vi "Main[Top VI].vi"() -> ()   [LabVIEW 2011]
uses:
  <vilib>/picture/picture.llb/imagedata.ctl
panel:
  out "Trate2":dbl caption="帧率T：" format="%#.1f"
  out "Rrate2":dbl caption="帧率R：" format="%#.1f"
  out "errcnt2":i32 caption="校验错误："
  out "Trate1":dbl caption="帧率T：" format="%#.1f"
  out "DevIndex":u32
  in  "path":path
  out "Rrate1":dbl caption="帧率R：" format="%#.1f"
  out "errcnt1":i32 caption="校验错误："
  in  "reciveEnable":bool=TRUE
  in  "ID Filter Set":bool
  in  "ID Filter Str":string="01 02"
  in  "ID Filter":enum32{"enable", "disable"}(radio)=enum."disable" caption="接收滤波ID设置(直接ID号)"
  in  "list":i32(listbox)
  in  "savefile":bool
  in  "sendfile":bool
  in  "clear":bool
  in  "send stop":bool
  out "SaveCnt":u32 caption="保存总帧数:"
  in  "ID Type":enum32{"left", "right"}(radio)=enum."right" caption="ID 格式"
  in  "Send":bool
  in  "Data Inc":bool
  in  "sendcycle":i32=10 caption="发送周期:" min=0 max=99999999 step=1
  in  "data":string="00 00 00 00 00 00 00 00" caption="数据:"
  in  "ID Inc":bool
  in  "SendCnt":i32=1 caption="发送总帧数:" min=-1
  in  "CAN Channel":enum16{"1", "2"}(ring) caption="CAN通道:"
  in  "Frame ID":string="00 00 00 01" caption="帧ID:"
  in  "Frame Type":enum16{"数据帧", "远程帧"}(ring) caption="帧类型:"
  in  "Frame Format":enum16{"标准帧", "扩展帧"}(ring) caption="帧格式:"
  # "ms"
  # "统计数据：通道2"
  # "统计数据：通道1"
  # "CAN发送"
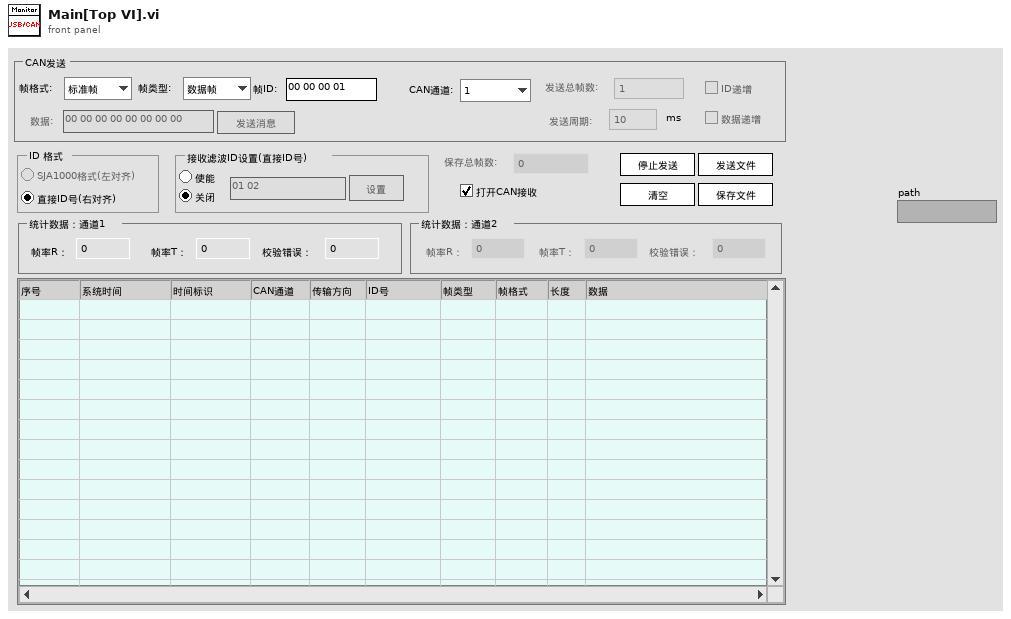
[diagram p1: front panel]
types:
  T1 = enum16{"Init", "RegistEvent", "run", "unRegistEvent", "Release", "Exit"}
  T2 = cluster{"type":u16, "scantime":u16, "highspd":bool, "disp":bool, "save":bool, "hl":bool, "ID合并":bool, "Rfun":u16, "Tfun":u16, "chk1":bool, "chk2":bool, "format":enum16{"hex", "dec", "oct", "bin"}, "rateR1":bool, "rateR2":bool, "rateT1":bool, "rateT2":bool, "RcvE1":bool, "RcvE2":bool, "TSFormat":enum16{"原始值", "实际值"}, "RcvLen":i16}
  T3 = typedef "imagedata.ctl" = cluster{"image type":i32, "image depth":i32, "image":u8[], "mask":u8[], "colors":u32[], "Rectangle":cluster{"left":i16, "top":i16, "right":i16, "bottom":i16}}
  T4 = enum8{"Enabled", "Disabled", "Disabled and Grayed Out"}
  T5 = typedef "Param.ctl" = cluster{"kCANBAUD":u8, "BTR0":u8, "BTR1":u8, "MODE":u8, "FILTER":u8, "ACR0":u32, "AMR0":u32, "FlashParam":u32, "BAUD":u32, "SJW":u8, "BRP":u8, "SAM":u8, "PHS2_SEL":u8, "PRSEG":u8, "PHSEG1":u8, "PHSEG2":u8}
  T6 = cluster{"hw_Version":u16, "fw_Version":u16, "dr_Version":u16, "in_Version":u16, "irq_Num":u16, "can_Num":u8, "str_Serial_Num":string, "str_hw_Type":string, "Reserved":u8[]}
  T7 = cluster{"hw_Version":u16, "fw_Version":u16, "dr_Version":u16, "in_Version":u16, "irq_Num":u16, "can_Num":u8, "reserved":u8, "str_Serial_Num":string, "str_hw_Type":string, "str_GYUsb_Serial":string[]}
  T8 = enum32{"Bad", "Idle", "Run top level", "Running"}
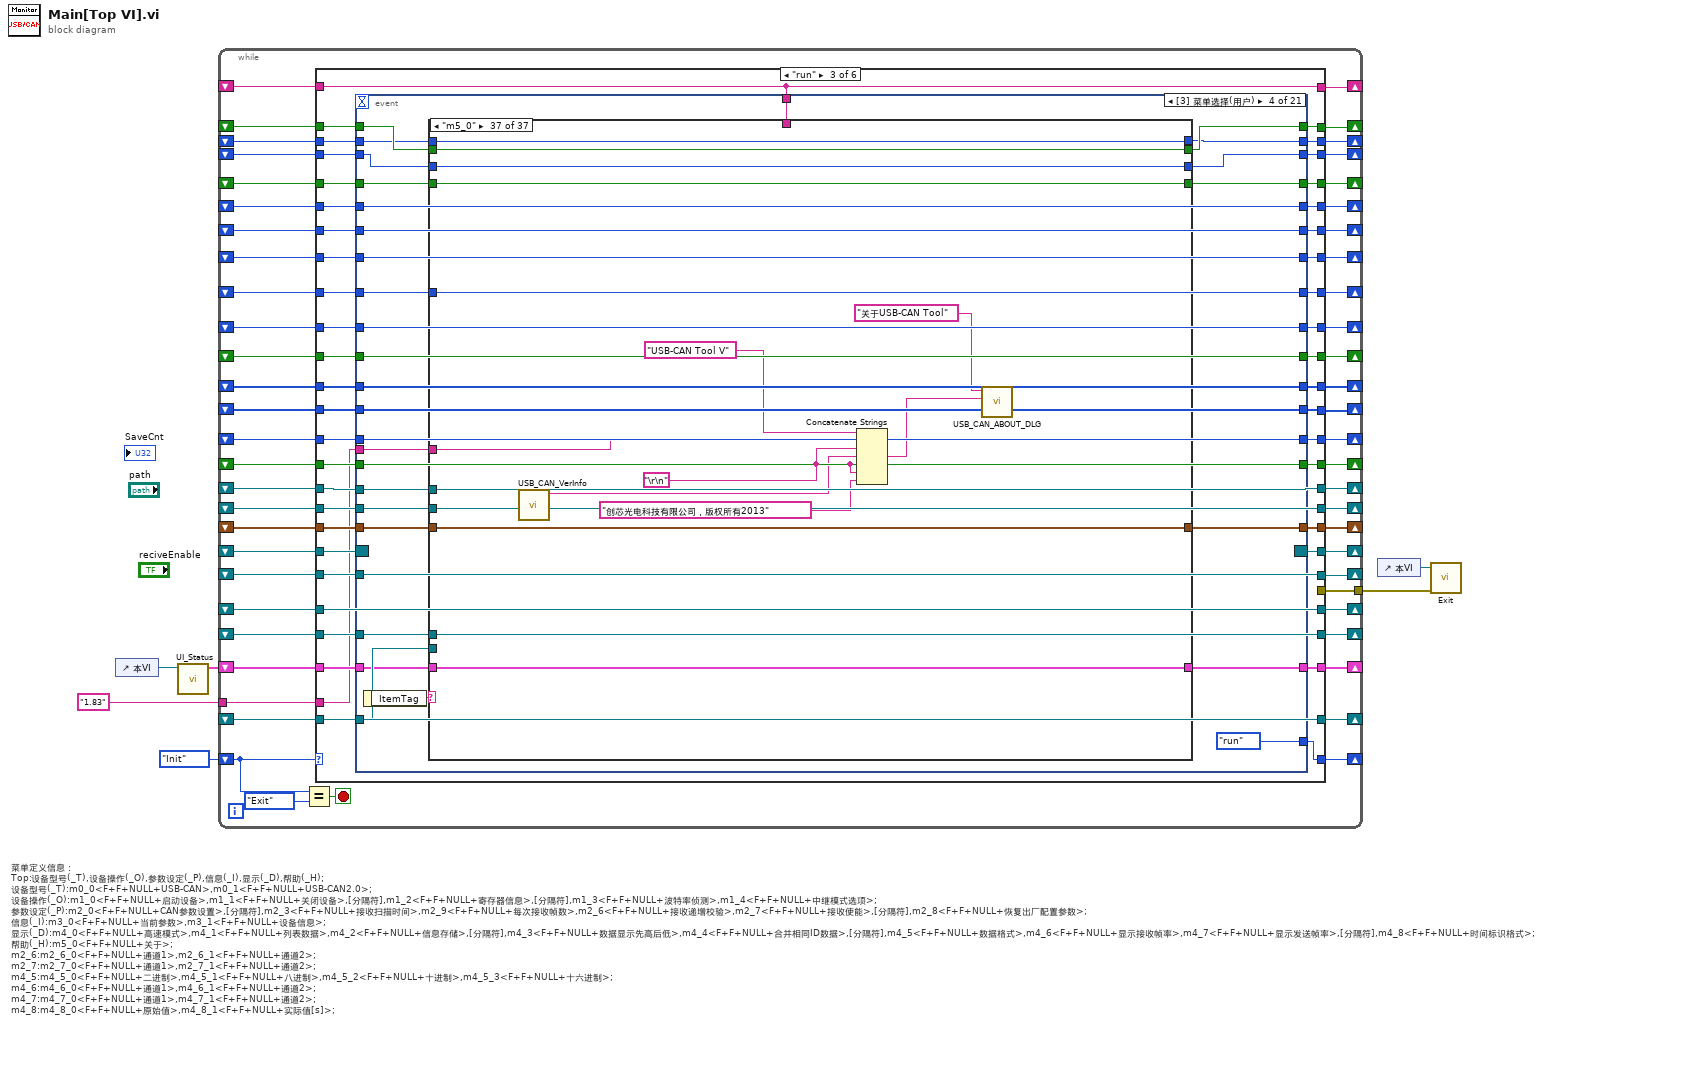
[diagram p0: block diagram]
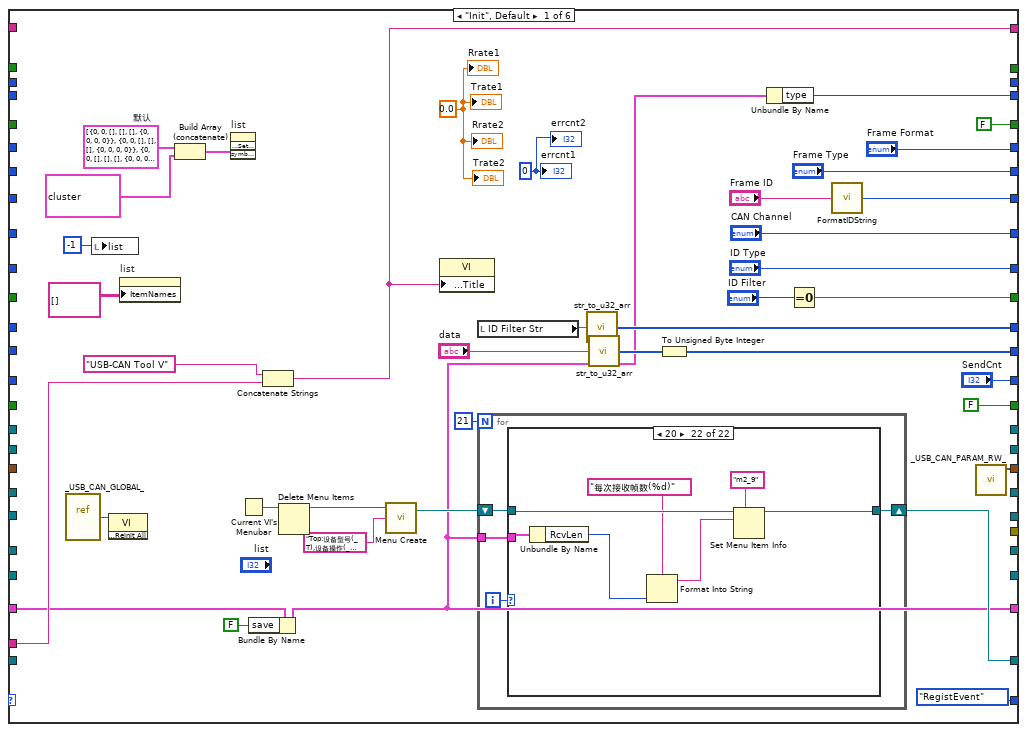
[diagram p2: hidden frame]
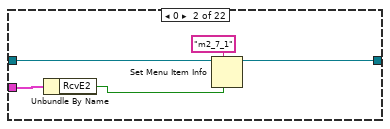
[diagram p4: hidden frame]
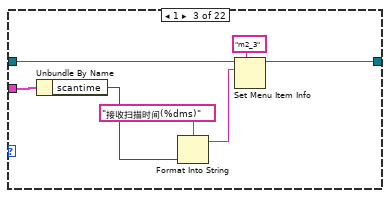
[diagram p5: hidden frame]
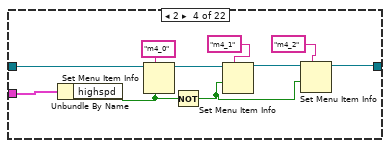
[diagram p6: hidden frame]
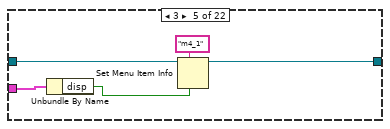
[diagram p7: hidden frame]
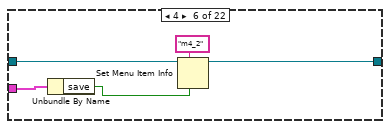
[diagram p8: hidden frame]
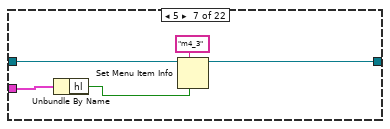
[diagram p9: hidden frame]
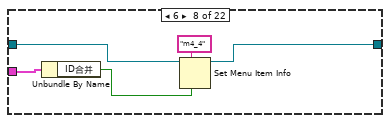
[diagram p10: hidden frame]
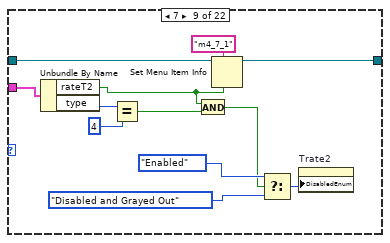
[diagram p11: hidden frame]
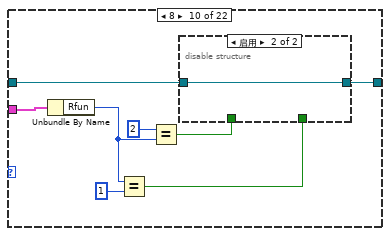
[diagram p12: hidden frame]
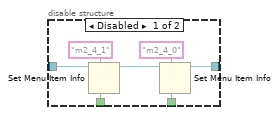
[diagram p13: hidden frame]
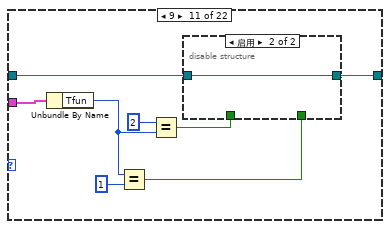
[diagram p14: hidden frame]
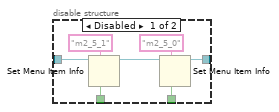
[diagram p15: hidden frame]
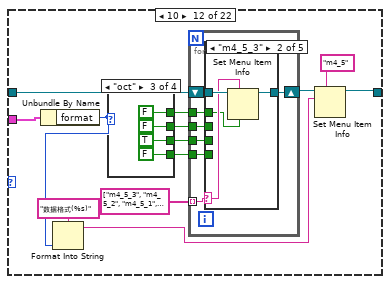
[diagram p16: hidden frame]
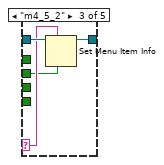
[diagram p18: hidden frame]
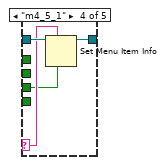
[diagram p19: hidden frame]
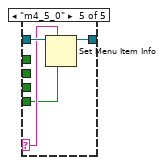
[diagram p20: hidden frame]
diagram:
  # "菜单定义信息：\nTop:设备型号(_T),设备操作(_O),参数设定(_P),信息(_I),显示(_D),帮助(_H);\n设备型号(_T):m0_0<F+F+NULL+USB-CAN>,m0_1<F+F+NULL+USB-CAN2.0>;\n设备操作(_O):m1_0<F+F+NULL+启动设备>,m1_1<F+F+NULL+关闭设备>,[分隔符],m1_2<F+F+NULL+寄存器信息>,[分隔符],m1_3<F+F+NULL+波特率侦测>,m1_4<F+F+NULL+中继模式选项>;\n参数设定(_P):m2_0<F+F+NULL+CAN参数设置>,[分隔符],m2_3<F+F+NULL+接收扫描时间>,m2_9<F+F+NULL+每次接收帧数>,m2_6<F+F+NULL+接收递增校验>,m2_7<F+F+NULL+接收使能>,[分隔符],m2_8<F+F+NULL+恢复出厂配置参数>;\n信息(_I):m3_0<F+F+NULL+当前参数>,m3_1<F+F+NULL+设备信息>;\n显示(_D):m4_0<F+F+NULL+高速模式>,m4_1<F+F+NULL+列表数据>,m4_2<F+F+NULL+信息存储>,[分隔符],m4_3<F+F+NULL+数据显示先高后低>,m4_4<F+F+NULL+合并相同ID数据>,[分隔符],m4_5<F+F+NULL+数据格式>,m4_6<F+F+NULL+显示接收帧率>,m4_7<F+F+NULL+显示发送帧率>,[分隔符],m4_8<F+F+NULL+时间标识格式>;\n帮助(_H):m5_0<F+F+NULL+关于>;\nm2_6:m2_6_0<F+F+NULL+通道1>,m2_6_1<F+F+NULL+通道2>;\nm2_7:m2_7_0<F+F+NULL+通道1>,m2_7_1<F+F+NULL+通道2>;\nm4_5:m4_5_0<F+F+NULL+二进制>,m4_5_1<F+F+NULL+八进制>,m4_5_2<F+F+NULL+十进制>,m4_5_3<F+F+NULL+十六进制>;\nm4_6:m4_6_0<F+F+NULL+通道1>,m4_6_1<F+F+NULL+通道2>;\nm4_7:m4_7_0<F+F+NULL+通道1>,m4_7_1<F+F+NULL+通道2>;\nm4_8:m4_8_0<F+F+NULL+原始值>,m4_8_1<F+F+NULL+实际值[s]>;"
  n1 = control-ref of="本VI"() -> (w5:refnum<vi>)
  n2 = call "UI_Status.vi"("VI ref"=w5) -> ("menu status in out"=w4:T2)  [unwired: 9 in, 1 out]
  n3 = while {
    shift-right: [w57] -> _
    shift-left: T1."Init" -> [w60]
    shift-right: [w56] -> _
    shift-left: _ -> [w55]
    shift-right: [w53] -> _
    shift-left: _ -> [w54]
    shift-right: [w52] -> _
    shift-left: _ -> [w51]
    shift-right: [w50] -> _
    shift-left: _ -> [w49]
    shift-right: [w48] -> _
    shift-left: _ -> [w47]
    shift-right: [w46] -> _
    shift-left: _ -> [w45]
    shift-right: [w44] -> _
    shift-left: _ -> [w43]
    shift-right: [w42] -> _
    shift-left: _ -> [w41]
    shift-right: [w40] -> _
    shift-left: _ -> [w39]
    shift-right: [w38] -> _
    shift-left: _ -> [w37]
    shift-right: [w36] -> _
    shift-left: _ -> [w35]
    shift-right: [w34] -> _
    shift-left: _ -> [w33]
    shift-right: [w31] -> _
    shift-left: _ -> [w32]
    shift-right: [w30] -> _
    shift-left: _ -> [w29]
    shift-right: [w28] -> _
    shift-left: _ -> [w27]
    shift-right: [w26] -> _
    shift-left: _ -> [w25]
    shift-right: [w24] -> _
    shift-left: _ -> [w22]
    shift-right: [w23] -> _
    shift-left: _ -> [w21]
    tunnel: [w20] -> w3
    shift-right: [w19] -> _
    shift-left: _ -> [w18]
    shift-right: [w17] -> _
    shift-left: w4 -> [w16]
    shift-right: [w15] -> _
    shift-left: _ -> [w14]
    shift-right: [w13] -> _
    shift-left: _ -> [w12]
    shift-right: [w11] -> _
    shift-left: _ -> [w10]
    shift-right: [w9] -> _
    shift-left: _ -> [w8]
    tunnel: "1.83" ("FileVersion") -> [w7]
    stop <- w58 stop-if-true
    n4 = Equal?(x=w60, y=T1."Exit") -> (x = y?=w58:bool)
    n5 = case shown="\"run\"" w60 {
      tunnel: [T1."RegistEvent" T1."run" w700 T1."Release" T1."Exit" T1."Exit"] -> w57
      tunnel: [FALSE w412 w710 _ _ _] -> w56
      tunnel: w55 -> [_ w412 w720 _ _ _]
      tunnel: w54 -> [_ w411 w719 _ _ _]
      tunnel: ["Frame Format" w411 w709 _ _ _] -> w53
      tunnel: ["Frame Type" w398 w708 _ _ _] -> w52
      tunnel: w51 -> [_ w398 w718 _ _ _]
      tunnel: [w94 w410 w707 _ _ _] -> w50
      tunnel: w49 -> [_ w410 w717 _ _ _]
      tunnel: ["CAN Channel" w397 w706 _ _ _] -> w48
      tunnel: w47 -> [_ w397 w716 _ _ _]
      tunnel: ["ID Type" w409 w705 _ _ _] -> w46
      tunnel: w45 -> [_ w409 w715 _ _ _]
      tunnel: [w64 w384 w703 _ _ _] -> w44
      tunnel: w43 -> [_ w384 w713 _ _ _]
      tunnel: [w90 w385 w704 _ _ _] -> w42
      tunnel: w41 -> [_ w385 w714 _ _ _]
      tunnel: [w81 w408 w702 _ _ _] -> w40
      tunnel: w39 -> [_ w408 w712 _ _ _]
      tunnel: ["SendCnt" w407 w701 _ _ _] -> w38
      tunnel: w37 -> [_ w407 w711 _ _ _]
      tunnel: [FALSE w406 w698 _ _ _] -> w36
      tunnel: w35 -> [_ w406 w699 _ _ _]
      tunnel: [w72 w405 w685 w2109 w2157 _] -> w34
      tunnel: w33 -> [_ w405 w685 w2109 w2157 _]
      tunnel: w32 -> [_ w404 w697 w2103 _ _]
      tunnel: [w66 w404 w696 _ _ _] -> w31
      tunnel: [_ w388 w695 _ _ _] -> w30
      tunnel: w29 -> [_ _ w695 w2127 _ _]
      tunnel: [_ w387 w694 _ _ _] -> w28
      tunnel: w27 -> [_ _ w694 w2120 _ _]
      tunnel: [w78 w399 w692 _ _ _] -> w26
      tunnel: w25 -> [_ w399 w693 w2111 _ _]
      tunnel: [_ w395 w690 _ _ _] -> w24
      tunnel: [_ w394 w689 _ _ _] -> w23
      tunnel: w22 -> [_ _ w691 w2117 _ _]
      tunnel: w21 -> [_ _ w689 w2115 _ _]
      tunnel: [_ _ _ w2114 _ _] -> w20
      tunnel: [_ w389 w688 _ _ _] -> w19
      tunnel: w18 -> [_ _ w688 w2112 _ _]
      tunnel: [w63 w380 w686 w2108 _ _] -> w17
      tunnel: w16 -> [w65 w380 w687 w2108 w2154 _]
      tunnel: [_ FALSE w683 _ _ _] -> w15
      tunnel: w14 -> [_ _ w684 _ _ _]
      tunnel: [_ w375 w682 _ _ _] -> w13
      tunnel: w12 -> [_ _ w682 w2106 _ _]
      tunnel: [_ _ w680 _ _ _] -> w11
      tunnel: w10 -> [_ _ w681 _ _ _]
      tunnel: [w69 w374 w679 w2105 w2153 w2163] -> w9
      tunnel: w8 -> [_ w374 w679 w2105 w2153 w2163]
      tunnel: w7 -> [w70 _ w678 _ _ _]
      frame "Init", Default {
        w67 = 0.0 ("rate")
        w77 = T3[] [{"image type"=0, "image depth"=0, "image"=[], "mask"=[], "colors"=[], "Rectangle"={"left"=0, "top"=0, "right"=0, "bottom"=0}}, {"image type"=0, "image depth"=0, "image"=[], "mask"=[], "colors"=[], "Rectangle"={"left"=0, "top"=0, "right"=0, "bottom"=0}}, {"image type"=0, "image depth"=0, "image"=[], "mask"=[], "colors"=[], "Rectangle"={"left"=0, "top"=0, "right"=0, "bottom"=0}}, {"image type"=0, "image depth"=0, "image"=[], "mask"=[], "colors"=[], "Rectangle"={"left"=0, "top"=0, "right"=0, "bottom"=0}}, {"image type"=0, "image depth"=0, "image"=[], "mask"=[], "colors"=[], "Rectangle"={"left"=0, "top"=0, "right"=0, "bottom"=0}}, {"image type"=0, "image depth"=0, "image"=[], "mask"=[], "colors"=[], "Rectangle"={"left"=0, "top"=0, "right"=0, "bottom"=0}}, {"image type"=0, "image depth"=0, "image"=[], "mask"=[], "colors"=[], "Rectangle"={"left"=0, "top"=0, "right"=0, "bottom"=0}}, {"image type"=0, "image depth"=0, "image"=[], "mask"=[], "colors"=[], "Rectangle"={"left"=0, "top"=0, "right"=0, "bottom"=0}}, {"image type"=0, "image depth"=0, "image"=[], "mask"=[], "colors"=[], "Rectangle"={"left"=0, "top"=0, "right"=0, "bottom"=0}}, {"image type"=0, "image depth"=0, "image"=[], "mask"=[], "colors"=[], "Rectangle"={"left"=0, "top"=0, "right"=0, "bottom"=0}}, {"image type"=0, "image depth"=0, "image"=[], "mask"=[], "colors"=[], "Rectangle"={"left"=0, "top"=0, "right"=0, "bottom"=0}}, {"image type"=0, "image depth"=0, "image"=[], "mask"=[], "colors"=[], "Rectangle"={"left"=0, "top"=0, "right"=0, "bottom"=0}}, {"image type"=0, "image depth"=0, "image"=[], "mask"=[], "colors"=[], "Rectangle"={"left"=0, "top"=0, "right"=0, "bottom"=0}}, {"image type"=0, "image depth"=0, "image"=[], "mask"=[], "colors"=[], "Rectangle"={"left"=0, "top"=0, "right"=0, "bottom"=0}}, {"image type"=0, "image depth"=0, "image"=[], "mask"=[], "colors"=[], "Rectangle"={"left"=0, "top"=0, "right"=0, "bottom"=0}}, {"image type"=0, "image depth"=0, "image"=[], "mask"=[], "colors"=[], "Rectangle"={"left"=0, "top"=0, "right"=0, "bottom"=0}}, {"image type"=0, "image depth"=0, "image"=[], "mask"=[], "colors"=[], "Rectangle"={"left"=0, "top"=0, "right"=0, "bottom"=0}}, {"image type"=0, "image depth"=0, "image"=[], "mask"=[], "colors"=[], "Rectangle"={"left"=0, "top"=0, "right"=0, "bottom"=0}}, {"image type"=0, "image depth"=0, "image"=[], "mask"=[], "colors"=[], "Rectangle"={"left"=0, "top"=0, "right"=0, "bottom"=0}}, {"image type"=0, "image depth"=0, "image"=[], "mask"=[], "colors"=[], "Rectangle"={"left"=0, "top"=0, "right"=0, "bottom"=0}}, {"image type"=0, "image depth"=0, "image"=[], "mask"=[], "colors"=[], "Rectangle"={"left"=0, "top"=0, "right"=0, "bottom"=0}}, {"image type"=0, "image depth"=0, "image"=[], "mask"=[], "colors"=[], "Rectangle"={"left"=0, "top"=0, "right"=0, "bottom"=0}}, {"image type"=0, "image depth"=0, "image"=[], "mask"=[], "colors"=[], "Rectangle"={"left"=0, "top"=0, "right"=0, "bottom"=0}}, {"image type"=0, "image depth"=0, "image"=[], "mask"=[], "colors"=[], "Rectangle"={"left"=0, "top"=0, "right"=0, "bottom"=0}}, {"image type"=0, "image depth"=0, "image"=[], "mask"=[], "colors"=[], "Rectangle"={"left"=0, "top"=0, "right"=0, "bottom"=0}}, {"image type"=0, "image depth"=0, "image"=[], "mask"=[], "colors"=[], "Rectangle"={"left"=0, "top"=0, "right"=0, "bottom"=0}}, {"image type"=0, "image depth"=0, "image"=[], "mask"=[], "colors"=[], "Rectangle"={"left"=0, "top"=0, "right"=0, "bottom"=0}}, {"image type"=0, "image depth"=0, "image"=[], "mask"=[], "colors"=[], "Rectangle"={"left"=0, "top"=0, "right"=0, "bottom"=0}}, {"image type"=0, "image depth"=0, "image"=[], "mask"=[], "colors"=[], "Rectangle"={"left"=0, "top"=0, "right"=0, "bottom"=0}}, {"image type"=0, "image depth"=0, "image"=[], "mask"=[], "colors"=[], "Rectangle"={"left"=0, "top"=0, "right"=0, "bottom"=0}}, {"image type"=0, "image depth"=0, "image"=[], "mask"=[], "colors"=[], "Rectangle"={"left"=0, "top"=0, "right"=0, "bottom"=0}}, {"image type"=0, "image depth"=0, "image"=[], "mask"=[], "colors"=[], "Rectangle"={"left"=0, "top"=0, "right"=0, "bottom"=0}}, {"image type"=0, "image depth"=0, "image"=[], "mask"=[], "colors"=[], "Rectangle"={"left"=0, "top"=0, "right"=0, "bottom"=0}}, {"image type"=0, "image depth"=0, "image"=[], "mask"=[], "colors"=[], "Rectangle"={"left"=0, "top"=0, "right"=0, "bottom"=0}}, {"image type"=0, "image depth"=0, "image"=[], "mask"=[], "colors"=[], "Rectangle"={"left"=0, "top"=0, "right"=0, "bottom"=0}}, {"image type"=0, "image depth"=0, "image"=[], "mask"=[], "colors"=[], "Rectangle"={"left"=0, "top"=0, "right"=0, "bottom"=0}}, {"image type"=0, "image depth"=0, "image"=[], "mask"=[], "colors"=[], "Rectangle"={"left"=0, "top"=0, "right"=0, "bottom"=0}}]  # 默认
        w68 = 0 ("errcnt")
        n6 = vi-ref "_USB_CAN_GLOBAL_.vi"() -> (w82:refnum<vi>)
        n7 = local write "list"(-1 ("list")) -> ()
        n8 = invoke class="VI" method="Default Vals.Reinit All"(reference=w82) -> ()  [unwired: 2 in, 3 out]
        n9 = property on="list" class="MCListbox (严格)"("ItemNames"=string[][] [] ("项名")) -> ()  [unwired: 2 in, 2 out]
        n10 = Build Array (concatenate)(w77, T3[] [{"image type"=0, "image depth"=32, "image"=array[1024 elements], "mask"=[255, 255, 255, 255, 255, 255, 255, 255, 255, 255, 255, 255, 255, 255, 255, 255, 255, 255, 255, 255, 255, 255, 255, 255, 255, 255, 255, 255, 255, 255, 255, 255], "colors"=[], "Rectangle"={"left"=0, "top"=0, "right"=16, "bottom"=16}}, {"image type"=0, "image depth"=32, "image"=array[1024 elements], "mask"=[255, 255, 255, 255, 255, 255, 255, 255, 255, 255, 255, 255, 255, 255, 255, 255, 255, 255, 255, 255, 255, 255, 255, 255, 255, 255, 255, 255, 255, 255, 255, 255], "colors"=[], "Rectangle"={"left"=0, "top"=0, "right"=16, "bottom"=16}}] ("数组")) -> (w76:T3[])
        n11 = invoke on="list" class="MCListbox (严格)" method="Custom Item Symbols.Set Symbol Array"("symbols"=w76) -> ()  [unwired: 3 in, 4 out]
        n12 = Current VI's Menubar() -> (w84:refnum<k9>)
        n13 = Bundle By Name(cluster=w65, "save"=FALSE) -> (w63:T2)
        n14 = Concatenate Strings("USB-CAN Tool V", w70) -> (w69:string)
        n15 = Delete Menu Items(9:w84) -> (3:w83:refnum<k9>)  [unwired: 1 in, 3 out]
        n16 = call "Menu Create.vi"("String"="Top:设备型号(_T),设备操作(_O),参数设定(_P),信息(_I),显示(_D),帮助(_H);\n设备型号(_T):m0_0<F+F+NULL+USB-CAN>,m0_1<F+F+NULL+USB-CAN2.0>;\n设备操作(_O):m1_0<F+F+NULL+启动设备>,m1_1<F+F+NULL+关闭设备>,[分隔符],m1_2<F+F+NULL+寄存器信息>,[分隔符],m1_3<F+F+NULL+波特率侦测>,m1_4<F+F+NULL+中继模式选项>;\n参数设定(_P):m2_0<F+F+NULL+CAN参数设置>,[分隔符],m2_3<F+F+NULL+接收扫描时间>,m2_9<F+F+NULL+每次接收帧数>,m2_6<F+F+NULL+接收递增校验>,m2_7<F+F+NULL+接收使能>,[分隔符],m2_8<F+F+NULL+恢复出厂配置参数>;\n信息(_I):m3_0<F+F+NULL+当前参数>,m3_1<F+F+NULL+设备信息>;\n显示(_D):m4_0<F+F+NULL+高速模式>,m4_1<F+F+NULL+列表数据>,m4_2<F+F+NULL+信息存储>,[分隔符],m4_3<F+F+NULL+数据显示先高后低>,m4_4<F+F+NULL+合并相同ID数据>,[分隔符],m4_5<F+F+NULL+数据格式>,m4_6<F+F+NULL+显示接收帧率>,m4_7<F+F+NULL+显示发送帧率>,[分隔符],m4_8<F+F+NULL+时间标识格式>;\n帮助(_H):m5_0<F+F+NULL+关于>;\nm2_6:m2_6_0<F+F+NULL+通道1>,m2_6_1<F+F+NULL+通道2>;\nm2_7:m2_7_0<F+F+NULL+通道1>,m2_7_1<F+F+NULL+通道2>;\nm4_5:m4_5_0<F+F+NULL+二进制>,m4_5_1<F+F+NULL+八进制>,m4_5_2<F+F+NULL+十进制>,m4_5_3<F+F+NULL+十六进制>;\nm4_6:m4_6_0<F+F+NULL+通道1>,m4_6_1<F+F+NULL+通道2>;\nm4_7:m4_7_0<F+F+NULL+通道1>,m4_7_1<F+F+NULL+通道2>;\nm4_8:m4_8_0<F+F+NULL+原始值>,m4_8_1<F+F+NULL+实际值[s]>;", "menubar in"=w83) -> ("menubar out"=w74:refnum<k9>)  [unwired: 1 in, 1 out]
        n17 = property class="VI"("Front Panel.Title"=w69) -> ()  [unwired: 2 in, 2 out]
        n18 = local read "ID Filter Str"() -> (w80:string)
        n19 = for {
          N: 21 -> [_]
          shift-right: [w100] -> w72
          shift-left: w74 -> [w101]
          tunnel: w63 -> [w102]
          i -> [w103]
          n20 = case shown="20" w103 {
            tunnel: w102 -> [_ w109 w116 w126 w131 w136 w141 w146 w158 w166 w182 w203 w251 w263 w271 w283 w291 w296 w313 _ w349 w359]
            tunnel: w101 -> [w104 w108 w115 w125 w130 w135 w140 w145 w157 w165 w181 w202 w250 w262 w270 w282 w290 w295 w311 w336 w355 w362]
            tunnel: [w104 w106 w114 w121 w129 w134 w139 w144 w155 w164 w180 w193 w248 w260 w268 w280 w288 w293 w310 w335 w351 w361] -> w100
            frame -1, Default {
            }
            frame 0 {
              n21 = Unbundle By Name(w109) -> ("RcvE2"=w105:bool)
              n22 = Set Menu Item Info(6:w105, 7:"m2_7_1" ("项标识符"), 11:w108) -> (3:w106:refnum<k9>)  [unwired: 4 in, 1 out]
            }
            frame 1 {
              n23 = Unbundle By Name(w116) -> ("scantime"=w112:u16)
              n24 = Format Into String(format string="接收扫描时间(%dms)" ("格式字符串"), w112) -> (resulting string=w110:string)  [unwired: 2 in, 1 out]
              n25 = Set Menu Item Info(7:"m2_3" ("项标识符"), 10:w110, 11:w115) -> (3:w114:refnum<k9>)  [unwired: 4 in, 1 out]
            }
            frame 2 {
              n26 = Unbundle By Name(w126) -> ("highspd"=w118:bool)
              n27 = Set Menu Item Info(6:w118, 7:"m4_0" ("项标识符"), 11:w125) -> (3:w123:refnum<k9>)  [unwired: 4 in, 1 out]
              n28 = Not(x=w118) -> (.not. x?=w117:bool)
              n29 = Set Menu Item Info(7:"m4_1" ("项标识符"), 9:w117, 11:w123) -> (3:w122:refnum<k9>)  [unwired: 4 in, 1 out]
              n30 = Set Menu Item Info(7:"m4_2" ("项标识符"), 9:w117, 11:w122) -> (3:w121:refnum<k9>)  [unwired: 4 in, 1 out]
            }
            frame 3 {
              n31 = Unbundle By Name(w131) -> ("disp"=w127:bool)
              n32 = Set Menu Item Info(6:w127, 7:"m4_1" ("项标识符"), 11:w130) -> (3:w129:refnum<k9>)  [unwired: 4 in, 1 out]
            }
            frame 4 {
              n33 = Unbundle By Name(w136) -> ("save"=w132:bool)
              n34 = Set Menu Item Info(6:w132, 7:"m4_2" ("项标识符"), 11:w135) -> (3:w134:refnum<k9>)  [unwired: 4 in, 1 out]
            }
            frame 5 {
              n35 = Unbundle By Name(w141) -> ("hl"=w137:bool)
              n36 = Set Menu Item Info(6:w137, 7:"m4_3" ("项标识符"), 11:w140) -> (3:w139:refnum<k9>)  [unwired: 4 in, 1 out]
            }
            frame 6 {
              n37 = Unbundle By Name(w146) -> ("ID合并"=w142:bool)
              n38 = Set Menu Item Info(6:w142, 7:"m4_4" ("项标识符"), 11:w145) -> (3:w144:refnum<k9>)  [unwired: 4 in, 1 out]
            }
            frame 7 {
              n39 = Unbundle By Name(w158) -> ("rateT2"=w149:bool, "type"=w151:u16)
              n40 = Equal?(x=w151, y=u16 4) -> (x = y?=w148:bool)
              n41 = And(x=w149, y=w148) -> (x .and. y?=w147:bool)
              n42 = Set Menu Item Info(6:w149, 7:"m4_7_1" ("项标识符"), 11:w157) -> (3:w155:refnum<k9>)  [unwired: 4 in, 1 out]
              n43 = Select(t=T4."Enabled" ("禁用"), s=w147, f=T4."Disabled and Grayed Out" ("禁用")) -> (s? t:f=w153:T4)
              n44 = property on="Trate2" class="DigNum (严格)"("DisabledEnum"=w153) -> ()  [unwired: 2 in, 2 out]
            }
            frame 8 {
              n45 = Unbundle By Name(w166) -> ("Rfun"=w161:u16)
              n46 = Equal?(x=w161, y=u16 1) -> (x = y?=w162:bool)
              n47 = Equal?(x=u16 2, y=w161) -> (x = y?=w159:bool)
              n48 = disable-structure shown="启用" {
                disable-tunnel: w165 -> [w173 w174]
                disable-tunnel: [w169 w174] -> w164
                disable-tunnel: w162 -> [w168 _]
                disable-tunnel: w159 -> [w167 _]
                frame Disabled {
                  n49 = Set Menu Item Info(6:w167, 7:"m2_4_1" ("项标识符"), 11:w173) -> (3:w170:refnum<k9>)  [unwired: 4 in, 1 out]
                  n50 = Set Menu Item Info(6:w168, 7:"m2_4_0" ("项标识符"), 11:w170) -> (3:w169:refnum<k9>)  [unwired: 4 in, 1 out]
                }
                frame Enabled {
                }
              }
            }
            frame 9 {
              n51 = Unbundle By Name(w182) -> ("Tfun"=w177:u16)
              n52 = Equal?(x=w177, y=u16 1) -> (x = y?=w178:bool)
              n53 = Equal?(x=u16 2, y=w177) -> (x = y?=w175:bool)
              n54 = disable-structure shown="启用" {
                disable-tunnel: w181 -> [w189 w190]
                disable-tunnel: [w185 w190] -> w180
                disable-tunnel: w178 -> [w184 _]
                disable-tunnel: w175 -> [w183 _]
                frame Disabled {
                  n55 = Set Menu Item Info(6:w183, 7:"m2_5_1" ("项标识符"), 11:w189) -> (3:w186:refnum<k9>)  [unwired: 4 in, 1 out]
                  n56 = Set Menu Item Info(6:w184, 7:"m2_5_0" ("项标识符"), 11:w186) -> (3:w185:refnum<k9>)  [unwired: 4 in, 1 out]
                }
                frame Enabled {
                }
              }
            }
            frame 10 {
              n57 = Unbundle By Name(w203) -> ("format"=w196:enum16{"hex", "dec", "oct", "bin"})
              n58 = Format Into String(format string="数据格式(%s)" ("格式字符串"), w196) -> (resulting string=w192:string)  [unwired: 2 in, 1 out]
              n59 = case shown="\"oct\"" w196 {
                tunnel: [TRUE FALSE FALSE FALSE] -> w201
                tunnel: [FALSE TRUE FALSE FALSE] -> w200
                tunnel: [FALSE FALSE TRUE FALSE] -> w199
                tunnel: [FALSE FALSE FALSE TRUE] -> w198
                frame "hex" {
                }
                frame "dec" {
                }
                frame "oct" {
                }
                frame "bin" {
                }
              }
              n60 = for {
                shift-right: [w209] -> w195
                shift-left: w202 -> [w210]
                tunnel: string[] ["m4_5_3", "m4_5_2", "m4_5_1", "m4_5_0"] -> [w208] mode=indexing
                tunnel: w201 -> [w207]
                tunnel: w200 -> [w206]
                tunnel: w199 -> [w205]
                tunnel: w198 -> [w204]
                n61 = case shown="\"m4_5_3\"" w208 {
                  selector: w208 -> [_ w213 w217 w221 w225]
                  tunnel: w210 -> [w211 w215 w219 w223 w227]
                  tunnel: [w211 w214 w218 w222 w226] -> w209
                  tunnel: w207 -> [_ w212 _ _ _]
                  tunnel: w206 -> [_ _ w216 _ _]
                  tunnel: w205 -> [_ _ _ w220 _]
                  tunnel: w204 -> [_ _ _ _ w224]
                  frame "假", Default {
                  }
                  frame "m4_5_3" {
                    n62 = Set Menu Item Info(6:w212, 7:w213, 11:w215) -> (3:w214:refnum<k9>)  [unwired: 4 in, 1 out]
                  }
                  frame "m4_5_2" {
                    n63 = Set Menu Item Info(6:w216, 7:w217, 11:w219) -> (3:w218:refnum<k9>)  [unwired: 4 in, 1 out]
                  }
                  frame "m4_5_1" {
                    n64 = Set Menu Item Info(6:w220, 7:w221, 11:w223) -> (3:w222:refnum<k9>)  [unwired: 4 in, 1 out]
                  }
                  frame "m4_5_0" {
                    n65 = Set Menu Item Info(6:w224, 7:w225, 11:w227) -> (3:w226:refnum<k9>)  [unwired: 4 in, 1 out]
                  }
                }
              }
              n66 = Set Menu Item Info(7:"m4_5" ("项标识符"), 10:w192, 11:w195) -> (3:w193:refnum<k9>)  [unwired: 4 in, 1 out]
            }
            frame 11 {
              n67 = Unbundle By Name(w251) -> ("chk1"=w244:bool)
              n68 = Set Menu Item Info(6:w244, 7:"m2_6_0" ("项标识符"), 11:w250) -> (3:w248:refnum<k9>)  [unwired: 4 in, 1 out]
              n69 = Select(t=T4."Enabled" ("禁用"), s=w244, f=T4."Disabled and Grayed Out" ("禁用")) -> (s? t:f=w246:T4)
              n70 = property on="errcnt1" class="DigNum (严格)"("DisabledEnum"=w246) -> ()  [unwired: 2 in, 2 out]
            }
            frame 12 {
              n71 = Unbundle By Name(w263) -> ("chk2"=w254:bool, "type"=w256:u16)
              n72 = Equal?(x=w256, y=u16 4) -> (x = y?=w253:bool)
              n73 = And(x=w254, y=w253) -> (x .and. y?=w252:bool)
              n74 = Set Menu Item Info(6:w254, 7:"m2_6_1" ("项标识符"), 11:w262) -> (3:w260:refnum<k9>)  [unwired: 4 in, 1 out]
              n75 = Select(t=T4."Enabled" ("禁用"), s=w252, f=T4."Disabled and Grayed Out" ("禁用")) -> (s? t:f=w258:T4)
              n76 = property on="errcnt2" class="DigNum (严格)"("DisabledEnum"=w258) -> ()  [unwired: 2 in, 2 out]
            }
            frame 13 {
              n77 = Unbundle By Name(w271) -> ("rateR1"=w264:bool)
              n78 = Set Menu Item Info(6:w264, 7:"m4_6_0" ("项标识符"), 11:w270) -> (3:w268:refnum<k9>)  [unwired: 4 in, 1 out]
              n79 = Select(t=T4."Enabled" ("禁用"), s=w264, f=T4."Disabled and Grayed Out" ("禁用")) -> (s? t:f=w266:T4)
              n80 = property on="Rrate1" class="DigNum (严格)"("DisabledEnum"=w266) -> ()  [unwired: 2 in, 2 out]
            }
            frame 14 {
              n81 = Unbundle By Name(w283) -> ("rateR2"=w274:bool, "type"=w276:u16)
              n82 = Equal?(x=w276, y=u16 4) -> (x = y?=w273:bool)
              n83 = And(x=w274, y=w273) -> (x .and. y?=w272:bool)
              n84 = Set Menu Item Info(6:w274, 7:"m4_6_1" ("项标识符"), 11:w282) -> (3:w280:refnum<k9>)  [unwired: 4 in, 1 out]
              n85 = Select(t=T4."Enabled" ("禁用"), s=w272, f=T4."Disabled and Grayed Out" ("禁用")) -> (s? t:f=w278:T4)
              n86 = property on="Rrate2" class="DigNum (严格)"("DisabledEnum"=w278) -> ()  [unwired: 2 in, 2 out]
            }
            frame 15 {
              n87 = Unbundle By Name(w291) -> ("rateT1"=w285:bool)
              n88 = Set Menu Item Info(6:w285, 7:"m4_7_0" ("项标识符"), 11:w290) -> (3:w288:refnum<k9>)  [unwired: 4 in, 1 out]
              n89 = Select(t=T4."Enabled" ("禁用"), s=w285, f=T4."Disabled and Grayed Out" ("禁用")) -> (s? t:f=w286:T4)
              n90 = property on="Trate1" class="DigNum (严格)"("DisabledEnum"=w286) -> ()  [unwired: 2 in, 2 out]
            }
            frame 16 {
              n91 = Unbundle By Name(w296) -> ("RcvE1"=w292:bool)
              n92 = Set Menu Item Info(6:w292, 7:"m2_7_0" ("项标识符"), 11:w295) -> (3:w293:refnum<k9>)  [unwired: 4 in, 1 out]
            }
            frame 17 {
              n93 = Unbundle By Name(w313) -> ("type"=w312:u16, "rateR2"=w300:bool, "rateT2"=w299:bool, "chk2"=w298:bool)
              n94 = case shown="3" w312 {
                tunnel: w311 -> [w316 w322 w334]
                tunnel: [w316 w319 w332] -> w306
                tunnel: [_ _ w331] -> w305
                tunnel: [w315 w318 w330] -> w302
                tunnel: [w315 w318 w328] -> w303
                tunnel: [w315 w318 w326] -> w301
                tunnel: w300 -> [_ _ w329]
                tunnel: w299 -> [_ _ w327]
                tunnel: w298 -> [_ _ w325]
                tunnel: [i32[] [1] ("禁用项[]") i32[] [1] ("禁用项[]") _] -> w297
                frame Default {
                  w315 = 2
                }
                frame 3 {
                  w318 = 2
                  n95 = Set Menu Item Info(6:TRUE ("已勾选"), 7:"m0_0" ("项标识符"), 11:w322) -> (3:w319:refnum<k9>)  [unwired: 4 in, 1 out]
                }
                frame 4 {
                  w323 = 2
                  w324 = 0
                  w331 = TRUE ("已勾选")
                  n96 = Set Menu Item Info(6:w331, 7:"m0_1" ("项标识符"), 11:w334) -> (3:w332:refnum<k9>)  [unwired: 4 in, 1 out]
                  n97 = Select(t=w324, s=w327, f=w323) -> (s? t:f=w328:i32)
                  n98 = Select(t=w324, s=w329, f=w323) -> (s? t:f=w330:i32)
                  n99 = Select(t=w324, s=w325, f=w323) -> (s? t:f=w326:i32)
                }
              }
              n100 = property on="CAN Channel" class="Enum (严格)"("Disabled Items []"=w297) -> ()  [unwired: 2 in, 2 out]
              n101 = property on="Trate2" class="DigNum (严格)"("DisabledEnum"=w303) -> ()  [unwired: 2 in, 2 out]
              n102 = property on="Rrate2" class="DigNum (严格)"("DisabledEnum"=w302) -> ()  [unwired: 2 in, 2 out]
              n103 = property on="errcnt2" class="DigNum (严格)"("DisabledEnum"=w301) -> ()  [unwired: 2 in, 2 out]
              n104 = Set Menu Item Info(7:"m2_6_1" ("项标识符"), 9:w305, 11:w306) -> (3:w310:refnum<k9>)  [unwired: 4 in, 1 out]
              n105 = Set Menu Item Info(7:"m2_7_1" ("项标识符"), 9:w305, 11:w306) -> ()  [unwired: 4 in, 2 out]
              n106 = Set Menu Item Info(7:"m4_6_1" ("项标识符"), 9:w305, 11:w306) -> ()  [unwired: 4 in, 2 out]
              n107 = Set Menu Item Info(7:"m4_7_1" ("项标识符"), 9:w305, 11:w306) -> ()  [unwired: 4 in, 2 out]
            }
            frame 18 {
              n108 = disable-structure shown="启用" {
                disable-tunnel: w336 -> [w343 w344]
                disable-tunnel: [w339 w344] -> w335
                frame Disabled {
                  w337 = FALSE ("已启用")
                  n109 = Set Menu Item Info(7:"m2_4" ("项标识符"), 9:w337, 11:w343) -> (0:w340:errorcluster, 3:w341:refnum<k9>)  [unwired: 4 in]
                  n110 = Set Menu Item Info(7:"m2_5" ("项标识符"), 8:w340, 9:w337, 11:w341) -> (3:w339:refnum<k9>)  [unwired: 3 in, 1 out]
                }
                frame Enabled {
                }
              }
            }
            frame 19 {
              n111 = Unbundle By Name(w349) -> ("TSFormat"=w348:enum16{"原始值", "实际值"})
              n112 = Equal?(x=w348, y=enum16{"原始值", "实际值"}."原始值") -> (x = y?=w346:bool)
              n113 = Set Menu Item Info(6:w346, 7:"m4_8_0" ("项标识符"), 11:w355) -> (0:w352:errorcluster, 3:w353:refnum<k9>)  [unwired: 4 in]
              n114 = Not(x=w346) -> (.not. x?=w345:bool)
              n115 = Set Menu Item Info(6:w345, 7:"m4_8_1" ("项标识符"), 8:w352, 11:w353) -> (3:w351:refnum<k9>)  [unwired: 3 in, 1 out]
            }
            frame 20 {
              n116 = Unbundle By Name(w359) -> ("RcvLen"=w358:i16)
              n117 = Format Into String(format string="每次接收帧数(%d)" ("格式字符串"), w358) -> (resulting string=w356:string)  [unwired: 2 in, 1 out]
              n118 = Set Menu Item Info(7:"m2_9" ("项标识符"), 10:w356, 11:w362) -> (3:w361:refnum<k9>)  [unwired: 4 in, 1 out]
            }
          }
        }
        n119 = call "str_to_u32_arr.vi"("string"=w80) -> ("array"=w64:u32[])
        n120 = call "str_to_u32_arr.vi"("string"="data") -> ("array"=w85:u32[])
        n121 = To Unsigned Byte Integer(number=w85) -> (unsigned 8bit integer=w81:u8[])
        n122 = Unbundle By Name(w63) -> ("type"=w66:u16)
        n123 = Equal To 0?(x="ID Filter") -> (x = 0?=w90:bool)
        n124 = call "FormatIDString.vi"("ID String"="Frame ID") -> ("ID"=w94:u32)
        n125 = call "_USB_CAN_PARAM_RW_.vi"() -> ("param out"=w78:T5[])  [unwired: 11 in]
        "errcnt1" <- w68
        "Rrate1" <- w67
        "Trate1" <- w67
        "errcnt2" <- w68
        "Rrate2" <- w67
        "Trate2" <- w67
      }
      frame "RegistEvent" {
        w376 = TRUE  # openCan
        w393 = TRUE  # savecancel
        w396 = TRUE  # sendover
        n126 = local read "reciveEnable"() -> (w372:bool)
        n127 = Unbundle By Name(w380) -> ("Rfun"=w379:u16, "Tfun"=w373:u16, "hl"=w371:bool, "scantime"=w367:u16)
        n128 = Open VI Reference(vi path=path "DeviceOP/ReciveThread.vi" ("VI路径")) -> (vi reference=w382:refnum<vi>, error out=w378:errorcluster)  [unwired: 5 in]
        n129 = global write "_USB_CAN_GLOBAL_.vi" "R-Enb"(w372) -> ()
        n130 = invoke class="VI" method="Ctrl Val.Set"(reference=w382, error in=w378, "Control Name"="RFun" ("控件名"), "Value"=w379) -> (reference out=w370:refnum<vi>, error out=w369:errorcluster)  [unwired: 1 in, 3 out]
        n131 = global write "_USB_CAN_GLOBAL_.vi" "Disp-HL"(w371) -> ()
        n132 = Open VI Reference(vi path=path "VIs/UpdateCANData.vi" ("VI路径"), options=0 ("选项")) -> (vi reference=w392:refnum<vi>, error out=w391:errorcluster)  [unwired: 4 in]
        n133 = Open VI Reference(vi path=path "VIs/CAN_DEBUG_Send.vi" ("VI路径")) -> (vi reference=w401:refnum<vi>, error out=w400:errorcluster)  [unwired: 5 in]
        n134 = invoke class="VI" method="Ctrl Val.Set"(reference=w370, error in=w369, "Control Name"="Scan time" ("控件名"), "Value"=w367) -> (reference out=w364:refnum<vi>, error out=w363:errorcluster)  [unwired: 1 in, 3 out]
        n135 = Create User Event(user event datatype=w393) -> (user event=w389:refnum<user-event>)  [unwired: 1 in, 1 out]
        n136 = for {
          N: 27 -> [_]
          shift-right: [w502] -> w388
          shift-left: w392 -> [w504]
          shift-right: [w501] -> _
          shift-left: w391 -> [w503]
          tunnel: w389 -> [w500]
          tunnel: w380 -> [w499]
          tunnel: w385 -> [w498]
          tunnel: w384 -> [w497]
          i -> [w505]
          n137 = case shown="25" w505 {
            tunnel: w504 -> [w507 w511 w517 w522 w529 w535 w541 w547 w554 w561 w568 w575 w581 w587 w593 w599 w606 w611 w618 w624 w630 w637 w644 w651 w658 w665 w672 w677]
            tunnel: w503 -> [w506 w510 w516 w520 w527 w534 w540 w546 w553 w560 w567 w574 w580 w586 w592 w598 w605 w609 w617 w623 w629 w636 w643 w650 w657 w664 w671 w676]
            tunnel: [w507 w508 w515 w519 w528 w533 w539 w545 w552 w559 w566 w573 w579 w585 w591 w597 w604 w608 w616 w622 w628 w635 w642 w649 w656 w663 w670 w675] -> w502
            tunnel: [w506 w509 w514 w518 w526 w532 w538 w544 w551 w558 w565 w572 w578 w584 w590 w596 w603 w607 w615 w621 w627 w634 w641 w648 w655 w662 w669 w674] -> w501
            tunnel: w500 -> [_ _ _ _ _ _ w536 _ _ _ _ _ _ _ _ _ _ _ _ _ _ _ _ _ _ _ _ _]
            tunnel: w499 -> [_ _ _ _ _ _ _ _ w549 w556 w563 w570 _ _ _ _ w601 _ _ _ _ w632 w639 w646 w653 w660 w667 _]
            tunnel: w498 -> [_ _ _ _ _ _ _ _ _ _ _ _ _ _ w588 _ _ _ _ _ _ _ _ _ _ _ _ _]
            tunnel: w497 -> [_ _ _ _ _ _ _ _ _ _ _ _ _ _ _ w594 _ _ _ _ _ _ _ _ _ _ _ _]
            frame -1, Default {
            }
            frame 0 {
              n138 = invoke class="VI" method="Default Vals.Reinit All"(reference=w511, error in=w510) -> (reference out=w508:refnum<vi>, error out=w509:errorcluster)  [unwired: 1 in, 1 out]
            }
            frame 1 {
              n139 = control-ref of="list"() -> (w512:refnum<vi>)
              n140 = invoke class="VI" method="Ctrl Val.Set"(reference=w517, error in=w516, "Control Name"="list ref" ("控件名"), "Value"=w512) -> (reference out=w515:refnum<vi>, error out=w514:errorcluster)  [unwired: 1 in, 3 out]
            }
            frame 2 {
              n141 = control-ref of="errcnt1"() -> (w521:refnum<vi>)
              n142 = invoke class="VI" method="Ctrl Val.Set"(reference=w522, error in=w520, "Control Name"="errcnt1" ("控件名"), "Value"=w521) -> (reference out=w519:refnum<vi>, error out=w518:errorcluster)  [unwired: 1 in, 3 out]
            }
            frame 3 {
              n143 = control-ref of="本VI"() -> (w524:refnum<vi>)
              n144 = invoke class="VI" method="Ctrl Val.Set"(reference=w529, error in=w527, "Control Name"="vi ref" ("控件名"), "Value"=w524) -> (reference out=w528:refnum<vi>, error out=w526:errorcluster)  [unwired: 1 in, 3 out]
            }
            frame 4 {
              n145 = control-ref of="Rrate1"() -> (w530:refnum<vi>)
              n146 = invoke class="VI" method="Ctrl Val.Set"(reference=w535, error in=w534, "Control Name"="rate0" ("控件名"), "Value"=w530) -> (reference out=w533:refnum<vi>, error out=w532:errorcluster)  [unwired: 1 in, 3 out]
            }
            frame 5 {
              n147 = invoke class="VI" method="Ctrl Val.Set"(reference=w541, error in=w540, "Control Name"="cancelEvt" ("控件名"), "Value"=w536) -> (reference out=w539:refnum<vi>, error out=w538:errorcluster)  [unwired: 1 in, 3 out]
            }
            frame 6 {
              n148 = control-ref of="path"() -> (w542:refnum<vi>)
              n149 = invoke class="VI" method="Ctrl Val.Set"(reference=w547, error in=w546, "Control Name"="path" ("控件名"), "Value"=w542) -> (reference out=w545:refnum<vi>, error out=w544:errorcluster)  [unwired: 1 in, 3 out]
            }
            frame 7 {
              n150 = Unbundle By Name(w549) -> ("chk1"=w548:bool)
              n151 = invoke class="VI" method="Ctrl Val.Set"(reference=w554, error in=w553, "Control Name"="check1" ("控件名"), "Value"=w548) -> (reference out=w552:refnum<vi>, error out=w551:errorcluster)  [unwired: 1 in, 3 out]
            }
            frame 8 {
              n152 = Unbundle By Name(w556) -> ("highspd"=w555:bool)
              n153 = invoke class="VI" method="Ctrl Val.Set"(reference=w561, error in=w560, "Control Name"="highspd" ("控件名"), "Value"=w555) -> (reference out=w559:refnum<vi>, error out=w558:errorcluster)  [unwired: 1 in, 3 out]
            }
            frame 9 {
              n154 = Unbundle By Name(w563) -> ("disp"=w562:bool)
              n155 = invoke class="VI" method="Ctrl Val.Set"(reference=w568, error in=w567, "Control Name"="disp" ("控件名"), "Value"=w562) -> (reference out=w566:refnum<vi>, error out=w565:errorcluster)  [unwired: 1 in, 3 out]
            }
            frame 10 {
              n156 = Unbundle By Name(w570) -> ("save"=w569:bool)
              n157 = invoke class="VI" method="Ctrl Val.Set"(reference=w575, error in=w574, "Control Name"="save" ("控件名"), "Value"=w569) -> (reference out=w573:refnum<vi>, error out=w572:errorcluster)  [unwired: 1 in, 3 out]
            }
            frame 11 {
              n158 = local read "reciveEnable"() -> (w576:bool)
              n159 = invoke class="VI" method="Ctrl Val.Set"(reference=w581, error in=w580, "Control Name"="Enable" ("控件名"), "Value"=w576) -> (reference out=w579:refnum<vi>, error out=w578:errorcluster)  [unwired: 1 in, 3 out]
            }
            frame 12 {
              n160 = control-ref of="SaveCnt"() -> (w582:refnum<vi>)
              n161 = invoke class="VI" method="Ctrl Val.Set"(reference=w587, error in=w586, "Control Name"="SaveCnt" ("控件名"), "Value"=w582) -> (reference out=w585:refnum<vi>, error out=w584:errorcluster)  [unwired: 1 in, 3 out]
            }
            frame 13 {
              n162 = invoke class="VI" method="Ctrl Val.Set"(reference=w593, error in=w592, "Control Name"="UseFilter" ("控件名"), "Value"=w588) -> (reference out=w591:refnum<vi>, error out=w590:errorcluster)  [unwired: 1 in, 3 out]
            }
            frame 14 {
              n163 = invoke class="VI" method="Ctrl Val.Set"(reference=w599, error in=w598, "Control Name"="Filter" ("控件名"), "Value"=w594) -> (reference out=w597:refnum<vi>, error out=w596:errorcluster)  [unwired: 1 in, 3 out]
            }
            frame 15 {
              n164 = Unbundle By Name(w601) -> ("ID合并"=w600:bool)
              n165 = invoke class="VI" method="Ctrl Val.Set"(reference=w606, error in=w605, "Control Name"="ID合并" ("控件名"), "Value"=w600) -> (reference out=w604:refnum<vi>, error out=w603:errorcluster)  [unwired: 1 in, 3 out]
            }
            frame 16 {
              n166 = control-ref of="errcnt2"() -> (w610:refnum<vi>)
              n167 = invoke class="VI" method="Ctrl Val.Set"(reference=w611, error in=w609, "Control Name"="errcnt2" ("控件名"), "Value"=w610) -> (reference out=w608:refnum<vi>, error out=w607:errorcluster)  [unwired: 1 in, 3 out]
            }
            frame 17 {
              n168 = control-ref of="Rrate2"() -> (w613:refnum<vi>)
              n169 = invoke class="VI" method="Ctrl Val.Set"(reference=w618, error in=w617, "Control Name"="rate1" ("控件名"), "Value"=w613) -> (reference out=w616:refnum<vi>, error out=w615:errorcluster)  [unwired: 1 in, 3 out]
            }
            frame 18 {
              n170 = control-ref of="Trate1"() -> (w619:refnum<vi>)
              n171 = invoke class="VI" method="Ctrl Val.Set"(reference=w624, error in=w623, "Control Name"="rate2" ("控件名"), "Value"=w619) -> (reference out=w622:refnum<vi>, error out=w621:errorcluster)  [unwired: 1 in, 3 out]
            }
            frame 19 {
              n172 = control-ref of="Trate2"() -> (w625:refnum<vi>)
              n173 = invoke class="VI" method="Ctrl Val.Set"(reference=w630, error in=w629, "Control Name"="rate3" ("控件名"), "Value"=w625) -> (reference out=w628:refnum<vi>, error out=w627:errorcluster)  [unwired: 1 in, 3 out]
            }
            frame 20 {
              n174 = Unbundle By Name(w632) -> ("chk2"=w631:bool)
              n175 = invoke class="VI" method="Ctrl Val.Set"(reference=w637, error in=w636, "Control Name"="check2" ("控件名"), "Value"=w631) -> (reference out=w635:refnum<vi>, error out=w634:errorcluster)  [unwired: 1 in, 3 out]
            }
            frame 21 {
              n176 = Unbundle By Name(w639) -> ("rateR1"=w638:bool)
              n177 = invoke class="VI" method="Ctrl Val.Set"(reference=w644, error in=w643, "Control Name"="Rrate1" ("控件名"), "Value"=w638) -> (reference out=w642:refnum<vi>, error out=w641:errorcluster)  [unwired: 1 in, 3 out]
            }
            frame 22 {
              n178 = Unbundle By Name(w646) -> ("rateR2"=w645:bool)
              n179 = invoke class="VI" method="Ctrl Val.Set"(reference=w651, error in=w650, "Control Name"="Rrate2" ("控件名"), "Value"=w645) -> (reference out=w649:refnum<vi>, error out=w648:errorcluster)  [unwired: 1 in, 3 out]
            }
            frame 23 {
              n180 = Unbundle By Name(w653) -> ("rateT1"=w652:bool)
              n181 = invoke class="VI" method="Ctrl Val.Set"(reference=w658, error in=w657, "Control Name"="Trate1" ("控件名"), "Value"=w652) -> (reference out=w656:refnum<vi>, error out=w655:errorcluster)  [unwired: 1 in, 3 out]
            }
            frame 24 {
              n182 = Unbundle By Name(w660) -> ("rateT2"=w659:bool)
              n183 = invoke class="VI" method="Ctrl Val.Set"(reference=w665, error in=w664, "Control Name"="Trate2" ("控件名"), "Value"=w659) -> (reference out=w663:refnum<vi>, error out=w662:errorcluster)  [unwired: 1 in, 3 out]
            }
            frame 26 {
              n184 = Unbundle By Name(w667) -> ("TSFormat"=w666:enum16{"原始值", "实际值"})
              n185 = invoke class="VI" method="Ctrl Val.Set"(reference=w672, error in=w671, "Control Name"="TSFormat" ("控件名"), "Value"=w666) -> (reference out=w670:refnum<vi>, error out=w669:errorcluster)  [unwired: 1 in, 3 out]
            }
            frame 25 {
              w673 = FALSE ("结束前等待")
              n186 = invoke class="VI" method="Run VI"(reference=w677, error in=w676, "Wait until done"=w673, "Auto Dispose Ref"=w673) -> (reference out=w675:refnum<vi>, error out=w674:errorcluster)  [unwired: 1 in, 3 out]
            }
          }
        }
        n187 = Close Reference(reference=w364, error in (no error)=w363) -> ()  [unwired: 1 out]
        n188 = Create User Event(user event datatype=w396) -> (user event=w394:refnum<user-event>)  [unwired: 1 in, 1 out]
        n189 = for {
          N: 12 -> [_]
          tunnel: w394 -> [w415]
          shift-right: [w418] -> w387
          shift-left: w401 -> [w419]
          shift-right: [w416] -> _
          shift-left: w400 -> [w417]
          tunnel: w373 -> [w414]
          i -> [w420]
          n190 = case shown="11" w420 {
            tunnel: w419 -> [w422 w426 w431 w437 w443 w449 w455 w461 w468 w475 w482 w490 w496]
            tunnel: [w422 w423 w428 w434 w440 w446 w452 w458 w465 w472 w479 w487 w493] -> w418
            tunnel: w417 -> [w421 w425 w430 w436 w442 w448 w454 w460 w467 w474 w481 w489 w495]
            tunnel: [w421 w424 w429 w435 w441 w447 w453 w459 w466 w473 w480 w488 w494] -> w416
            tunnel: w415 -> [_ _ w427 _ _ _ _ _ _ _ _ _ _]
            tunnel: w414 -> [_ _ _ _ _ _ _ w457 _ _ _ _ _]
            frame -1, Default {
            }
            frame 0 {
              n191 = invoke class="VI" method="Default Vals.Reinit All"(reference=w426, error in=w425) -> (reference out=w423:refnum<vi>, error out=w424:errorcluster)  [unwired: 1 in, 1 out]
            }
            frame 1 {
              n192 = invoke class="VI" method="Ctrl Val.Set"(reference=w431, error in=w430, "Control Name"="event" ("控件名"), "Value"=w427) -> (reference out=w428:refnum<vi>, error out=w429:errorcluster)  [unwired: 1 in, 3 out]
            }
            frame 2 {
              n193 = local read "sendcycle"() -> (w433:i32)
              n194 = invoke class="VI" method="Ctrl Val.Set"(reference=w437, error in=w436, "Control Name"="Cycle" ("控件名"), "Value"=w433) -> (reference out=w434:refnum<vi>, error out=w435:errorcluster)  [unwired: 1 in, 3 out]
            }
            frame 3 {
              n195 = local read "SendCnt"() -> (w439:i32)
              n196 = invoke class="VI" method="Ctrl Val.Set"(reference=w443, error in=w442, "Control Name"="FrameCnt" ("控件名"), "Value"=w439) -> (reference out=w440:refnum<vi>, error out=w441:errorcluster)  [unwired: 1 in, 3 out]
            }
            frame 4 {
              n197 = local read "ID Inc"() -> (w445:bool)
              n198 = invoke class="VI" method="Ctrl Val.Set"(reference=w449, error in=w448, "Control Name"="ID Inc" ("控件名"), "Value"=w445) -> (reference out=w446:refnum<vi>, error out=w447:errorcluster)  [unwired: 1 in, 3 out]
            }
            frame 5 {
              n199 = local read "Data Inc"() -> (w451:bool)
              n200 = invoke class="VI" method="Ctrl Val.Set"(reference=w455, error in=w454, "Control Name"="Data Inc" ("控件名"), "Value"=w451) -> (reference out=w452:refnum<vi>, error out=w453:errorcluster)  [unwired: 1 in, 3 out]
            }
            frame 10 {
              n201 = invoke class="VI" method="Ctrl Val.Set"(reference=w461, error in=w460, "Control Name"="TFun" ("控件名"), "Value"=w457) -> (reference out=w458:refnum<vi>, error out=w459:errorcluster)  [unwired: 1 in, 3 out]
            }
            frame 6 {
              n202 = local read "Frame ID"() -> (w464:string)
              n203 = call "FormatIDString.vi"("ID String"=w464) -> ("ID"=w463:u32)
              n204 = invoke class="VI" method="Ctrl Val.Set"(reference=w468, error in=w467, "Control Name"="ID" ("控件名"), "Value"=w463) -> (reference out=w465:refnum<vi>, error out=w466:errorcluster)  [unwired: 1 in, 3 out]
            }
            frame 7 {
              n205 = local read "Frame Format"() -> (w471:enum16{"标准帧", "扩展帧"})
              n206 = Not Equal To 0?(x=w471) -> (x != 0?=w470:bool)
              n207 = invoke class="VI" method="Ctrl Val.Set"(reference=w475, error in=w474, "Control Name"="ExtFrame" ("控件名"), "Value"=w470) -> (reference out=w472:refnum<vi>, error out=w473:errorcluster)  [unwired: 1 in, 3 out]
            }
            frame 8 {
              n208 = local read "Frame Type"() -> (w478:enum16{"数据帧", "远程帧"})
              n209 = Not Equal To 0?(x=w478) -> (x != 0?=w477:bool)
              n210 = invoke class="VI" method="Ctrl Val.Set"(reference=w482, error in=w481, "Control Name"="remote" ("控件名"), "Value"=w477) -> (reference out=w479:refnum<vi>, error out=w480:errorcluster)  [unwired: 1 in, 3 out]
            }
            frame 9 {
              n211 = local read "data"() -> (w485:string)
              n212 = call "str_to_u32_arr.vi"("string"=w485) -> ("array"=w486:u32[])
              n213 = To Unsigned Byte Integer(number=w486) -> (unsigned 8bit integer=w484:u8[])
              n214 = invoke class="VI" method="Ctrl Val.Set"(reference=w490, error in=w489, "Control Name"="data" ("控件名"), "Value"=w484) -> (reference out=w487:refnum<vi>, error out=w488:errorcluster)  [unwired: 1 in, 3 out]
            }
            frame 11 {
              w492 = FALSE ("结束前等待")
              n215 = invoke class="VI" method="Run VI"(reference=w496, error in=w495, "Wait until done"=w492, "Auto Dispose Ref"=w492) -> (reference out=w493:refnum<vi>, error out=w494:errorcluster)  [unwired: 1 in, 3 out]
            }
          }
        }
        n216 = Create User Event(user event datatype=w376) -> (user event=w375:refnum<user-event>)  [unwired: 1 in, 1 out]
        n217 = register-events(w394, w389, w375) -> (reference out=w395:refnum<event-registration>)  [unwired: 2 in, 1 out]
        n218 = property on="send stop" class="Bool (严格)"("Val(Sgnl)"=TRUE ("值(信号)")) -> ()  [unwired: 2 in, 2 out]
      }
      frame "run" {
        n219 = event shown="[3] 菜单选择(用户)" {
          selector: w691 -> [_ _ _ _ _ _ _ _ _ _ _ _ _ _ _ _ _ _ _ _ _]
          dyn-events: [_ _ _ _ _ _ _ _ _ _ _ _ _ _ _ _ _ _ _ _ _] -> w690
          timeout: _ -> [_ _ _ _ _ _ _ _ _ _ _ _ _ _ _ _ _ _ _ _ _]
          tunnel: w720 -> [w737 w760 w779 w794 _ w1730 w1734 w1796 w1816 w1836 w1841 w1926 w1951 w1974 w1997 w2016 w2033 w2050 w2068 w2085 w2102]
          tunnel: w719 -> [w736 w759 w778 w809 w1669 w1729 w1748 w1795 w1815 w1835 w1854 w1925 w1950 w1973 w1996 w2015 w2032 w2049 w2067 w2084 _]
          tunnel: w718 -> [w735 w758 w777 w808 w1668 w1728 w1747 w1794 w1814 w1834 w1853 w1924 w1949 w1972 w1995 w2014 w2031 w2048 w2066 _ w2101]
          tunnel: w717 -> [w734 w757 w776 w807 w1667 w1727 w1746 w1793 w1813 w1833 w1843 w1923 w1948 w1971 w1994 w2013 w2030 w2047 _ w2083 w2100]
          tunnel: w716 -> [w733 w756 w775 w795 w1659 w1726 w1731 w1792 w1812 w1832 w1837 w1922 w1947 w1970 w1993 w2012 w2029 _ w2065 w2082 w2099]
          tunnel: w715 -> [w732 w755 w774 w806 w1666 w1725 w1745 w1791 w1811 w1831 w1852 w1921 w1946 w1969 _ w2011 w2028 w2046 w2064 w2081 w2098]
          tunnel: w714 -> [w731 w754 w773 w805 w1665 w1724 w1744 w1790 w1810 w1830 w1851 w1920 w1939 _ w1992 w2010 w2027 w2045 w2063 w2080 w2097]
          tunnel: w713 -> [w730 w753 w772 w804 w1664 w1723 w1743 w1789 w1809 w1829 w1850 w1919 w1942 w1957 w1991 w2009 w2026 w2044 w2062 w2079 w2096]
          tunnel: w712 -> [w729 w752 w771 w803 w1663 w1722 w1742 w1788 w1808 w1828 w1845 w1918 w1945 w1968 w1990 _ w2025 w2043 w2061 w2078 w2095]
          tunnel: w711 -> [w728 w751 w770 w802 w1662 w1721 w1741 w1787 w1807 w1827 w1844 w1917 w1944 w1967 w1989 w2008 _ w2042 w2060 w2077 w2094]
          tunnel: [w737 w760 w779 w793 w1658 w1730 w1734 w1796 w1816 w1836 w1841 w1926 w1951 w1974 w1997 w2016 w2033 w2050 w2068 w2085 w2102] -> w710
          tunnel: [w736 w759 w778 w809 w1669 w1729 w1748 w1795 w1815 w1835 w1854 w1925 w1950 w1973 w1996 w2015 w2032 w2049 w2067 w2084 w2092] -> w709
          tunnel: [w735 w758 w777 w808 w1668 w1728 w1747 w1794 w1814 w1834 w1853 w1924 w1949 w1972 w1995 w2014 w2031 w2048 w2066 w2075 w2101] -> w708
          tunnel: [w734 w757 w776 w807 w1667 w1727 w1746 w1793 w1813 w1833 w1843 w1923 w1948 w1971 w1994 w2013 w2030 w2047 w2057 w2083 w2100] -> w707
          tunnel: [w733 w756 w775 w795 w1659 w1726 w1731 w1792 w1812 w1832 w1837 w1922 w1947 w1970 w1993 w2012 w2029 w2040 w2065 w2082 w2099] -> w706
          tunnel: [w732 w755 w774 w806 w1666 w1725 w1745 w1791 w1811 w1831 w1852 w1921 w1946 w1969 w1987 w2011 w2028 w2046 w2064 w2081 w2098] -> w705
          tunnel: [w731 w754 w773 w805 w1665 w1724 w1744 w1790 w1810 w1830 w1851 w1920 w1939 w1955 w1992 w2010 w2027 w2045 w2063 w2080 w2097] -> w704
          tunnel: [w730 w753 w772 w804 w1664 w1723 w1743 w1789 w1809 w1829 w1850 w1919 w1937 w1957 w1991 w2009 w2026 w2044 w2062 w2079 w2096] -> w703
          tunnel: [w729 w752 w771 w803 w1663 w1722 w1742 w1788 w1808 w1828 w1845 w1918 w1945 w1968 w1990 w2001 w2025 w2043 w2061 w2078 w2095] -> w702
          tunnel: [w728 w751 w770 w802 w1662 w1721 w1741 w1787 w1807 w1827 w1844 w1917 w1944 w1967 w1989 w2008 w2023 w2042 w2060 w2077 w2094] -> w701
          tunnel: [T1."run" T1."run" T1."run" T1."run" T1."run" T1."unRegistEvent" T1."run" T1."run" T1."run" T1."run" T1."run" T1."run" T1."run" T1."run" T1."run" T1."run" T1."run" T1."run" T1."run" T1."run" T1."run"] -> w700
          tunnel: w699 -> [w726 w749 w768 w800 w1660 w1719 w1739 w1785 w1805 w1825 _ _ w1941 w1960 w1986 w2006 w2022 w2039 w2056 w2074 w2091]
          tunnel: [w726 w749 w768 w800 w1660 w1719 w1739 w1785 w1805 w1825 TRUE FALSE w1941 w1960 w1986 w2006 w2022 w2039 w2056 w2074 w2091] -> w698
          tunnel: w685 -> [_ w745 _ w791 _ _ _ w1774 _ _ _ _ _ _ _ _ _ _ _ _ _]
          tunnel: w697 -> [w725 w748 w767 w799 w1647 w1717 w1738 w1784 w1804 w1824 w1847 w1912 w1940 w1959 w1985 w2005 w2021 w2038 w2055 w2073 w2090]
          tunnel: [w725 w748 w767 w798 w1647 w1717 w1738 w1784 w1804 w1824 w1847 w1912 w1940 w1959 w1985 w2005 w2021 w2038 w2055 w2073 w2090] -> w696
          tunnel: w695 -> [_ w746 _ w792 _ _ _ w1778 w1802 w1823 _ _ w1932 w1958 _ _ _ _ _ _ _]
          tunnel: w694 -> [_ _ _ w781 _ _ w1736 _ _ _ w1846 w1909 _ _ _ _ _ _ _ _ _]
          tunnel: w693 -> [w724 w738 w766 w797 w1651 w1716 w1737 w1783 w1800 w1822 w1842 w1911 w1936 w1956 w1984 w2004 w2020 w2037 w2054 w2072 w2089]
          tunnel: [w724 w738 w766 w796 w1649 w1716 w1737 w1783 w1800 w1822 w1842 w1911 w1936 w1956 w1984 w2004 w2020 w2037 w2054 w2072 w2089] -> w692
          tunnel: w689 -> [_ _ _ _ _ _ _ _ _ _ _ _ _ _ _ _ _ _ _ _ _]
          tunnel: w687 -> [w723 w743 w763 w789 w1650 w1715 w1735 w1776 w1799 w1821 w1840 w1908 w1930 w1954 w1983 w2000 w2019 w2036 w2053 w2071 w2088]
          tunnel: [w723 w741 w763 w788 w1650 w1715 w1735 w1775 w1799 w1821 w1840 w1908 w1930 w1954 w1983 w2000 w2019 w2036 w2053 w2071 w2088] -> w686
          tunnel: w684 -> [w722 w740 w762 w787 w1657 w1714 w1733 w1782 w1798 w1820 w1839 w1907 w1929 w1953 w1982 w1999 w2018 w2035 w2052 w2070 w2087]
          tunnel: [w722 w740 w762 w786 w1657 w1714 w1733 w1782 w1798 w1820 w1839 w1907 w1929 w1953 w1982 w1999 w2018 w2035 w2052 w2070 w2087] -> w683
          tunnel: w682 -> [_ _ _ w785 _ _ _ _ _ _ _ _ _ _ _ _ _ _ _ _ _]
          tunnel: w681 -> [w721 w739 w761 w784 w1644 w1713 w1732 w1781 w1797 w1819 w1838 w1906 w1928 w1952 w1981 w1998 w2017 w2034 w2051 w2069 w2086]
          tunnel: [w721 w739 w761 w783 w1648 w1713 w1732 w1781 w1797 w1819 w1838 w1906 w1928 w1952 w1981 w1998 w2017 w2034 w2051 w2069 w2086] -> w680
          tunnel: w679 -> [_ _ _ w782 w1653 _ _ _ _ _ _ _ _ _ _ _ _ _ _ _ _]
          tunnel: w678 -> [_ _ _ w780 _ _ _ _ _ _ _ _ _ _ _ _ _ _ _ _ _]
          event Timeout {
            n220 = event-data() -> ()  [unwired: 1 in, 1 out]
          }
          event User Event {
            w742 = FALSE
            n221 = event-data() -> ()  [unwired: 1 in, 1 out]
            n222 = Set Menu Item Info(6:w742, 7:"m4_2" ("项标识符"), 11:w745) -> ()  [unwired: 4 in, 2 out]
            n223 = invoke class="VI" method="Ctrl Val.Set"(reference=w746, "Control Name"="save" ("控件名"), "Value"=w742) -> ()  [unwired: 2 in, 5 out]
            n224 = Bundle By Name(cluster=w743, "save"=w742) -> (w741:T2)
          }
          event User Event {
            w764 = T4."Enabled" ("禁用")
            n225 = event-data() -> ()  [unwired: 1 in, 1 out]
            n226 = property on="send stop" class="Bool (严格)"("DisabledEnum"=T4."Disabled and Grayed Out" ("禁用")) -> ()  [unwired: 2 in, 2 out]
            n227 = property on="Send" class="Bool"("DisabledEnum"=w764) -> ()  [unwired: 2 in, 2 out]
            n228 = property on="data" class="Str"("DisabledEnum"=w764) -> ()  [unwired: 2 in, 2 out]
            n229 = property on="ID Inc" class="Bool (严格)"("DisabledEnum"=w764) -> ()  [unwired: 2 in, 2 out]
            n230 = property on="sendcycle" class="DigNum (严格)"("DisabledEnum"=w764) -> ()  [unwired: 2 in, 2 out]
            n231 = property on="Data Inc" class="Bool (严格)"("DisabledEnum"=w764) -> ()  [unwired: 2 in, 2 out]
            n232 = property on="SendCnt" class="DigNum (严格)"("DisabledEnum"=w764) -> ()  [unwired: 2 in, 2 out]
          }
          event Menu Selection (User) {
            n233 = event-data() -> ("ItemTag"=w790:string)  [unwired: 1 in]
            n234 = case shown="\"m5_0\"" w790 {
              selector: w790 -> [_ _ _ _ _ _ _ _ _ _ _ w1093 w1112 w1134 w1155 w1174 w1193 w1209 w1230 w1246 w1266 _ _ _ w1363 w1377 w1395 w1407 w1430 w1452 w1468 w1485 w1555 w1579 w1599 w1623 _]
              tunnel: w799 -> [w815 _ _ w889 w894 w925 w955 w975 w988 w1031 w1059 w1099 w1116 w1139 w1160 w1179 w1198 w1215 w1236 w1252 w1272 w1275 w1314 w1339 w1368 w1382 w1400 w1412 w1434 w1456 w1473 w1497 w1561 w1585 w1605 w1629 w1642]
              tunnel: [w815 u16 3 u16 4 w889 w894 w925 w955 w975 w988 w1031 w1059 w1099 w1116 w1139 w1160 w1179 w1198 w1215 w1236 w1252 w1272 w1275 w1314 w1339 w1368 w1382 w1400 w1412 w1434 w1456 w1473 w1497 w1561 w1585 w1605 w1629 w1642] -> w798
              tunnel: w797 -> [w814 w845 w881 w888 w896 w927 w957 w978 w990 w1032 w1061 w1101 w1118 w1137 w1158 w1177 w1196 w1213 w1234 w1250 w1270 w1276 w1321 w1341 w1367 w1381 w1399 w1411 w1433 w1455 w1472 w1496 w1559 w1583 w1603 w1627 w1641]
              tunnel: [w814 w845 w881 w888 w896 w927 w957 w978 w989 w1032 w1061 w1101 w1118 w1137 w1158 w1177 w1196 w1213 w1234 w1250 w1270 w1276 w1321 w1341 w1367 w1381 w1399 w1411 w1433 w1455 w1472 w1496 w1559 w1583 w1603 w1627 w1641] -> w796
              tunnel: w795 -> [_ _ _ _ _ _ _ _ _ w1030 _ _ _ _ _ _ _ _ _ _ _ _ _ _ _ _ _ _ _ _ _ _ _ _ _ _ _]
              tunnel: w794 -> [w813 w844 w880 w885 w895 w926 w956 _ w991 w1036 w1060 w1100 w1117 w1138 w1159 w1178 w1197 w1214 w1235 w1251 w1271 w1278 w1327 w1340 w1366 w1380 w1398 w1410 w1432 w1454 w1471 w1495 w1560 w1584 w1604 w1628 w1640]
              tunnel: [w813 w844 w880 w885 w890 w922 w952 _ w991 w1036 w1060 w1100 w1117 w1138 w1159 w1178 w1197 w1214 w1235 w1251 w1271 w1278 w1327 w1340 w1366 w1380 w1398 w1410 w1432 w1454 w1471 w1495 w1560 w1584 w1604 w1628 w1640] -> w793
              tunnel: w791 -> [_ w841 w875 _ _ _ _ _ _ _ _ w1094 w1113 w1135 w1156 w1175 w1194 w1210 w1231 w1247 w1267 _ _ _ w1365 w1379 w1397 w1409 w1431 w1453 w1470 w1486 w1556 w1580 w1600 w1624 _]
              tunnel: w792 -> [_ _ _ _ _ _ _ _ _ _ _ _ _ _ _ _ _ w1208 w1229 _ _ _ _ _ w1361 w1375 w1393 _ w1418 w1440 w1466 w1483 w1554 w1578 w1598 w1622 _]
              tunnel: w789 -> [w812 w828 w864 w887 w892 w924 w954 w977 w984 w1035 w1062 w1091 w1111 w1132 w1153 w1172 w1191 w1205 w1221 w1244 w1255 w1277 w1326 w1342 w1359 w1372 w1391 w1405 w1429 w1451 w1464 w1494 w1551 w1563 w1595 w1607 w1639]
              tunnel: [w812 w838 w874 w887 w892 w924 w954 w977 w984 w1035 w1062 w1090 w1110 w1133 w1154 w1173 w1192 w1206 w1227 w1245 w1265 w1277 w1326 w1342 w1358 w1371 w1390 w1404 w1428 w1450 w1462 w1493 w1552 w1576 w1596 w1620 w1639] -> w788
              tunnel: w787 -> [w811 w836 w872 _ _ _ _ w979 w987 w1034 w1058 w1098 w1115 w1127 w1148 w1170 w1189 w1204 w1226 w1243 w1264 w1279 w1324 w1338 w1357 w1370 w1389 w1403 w1427 w1449 w1461 w1492 w1550 w1575 w1594 w1619 w1637]
              tunnel: [w811 w836 w872 TRUE w890 w922 w952 w979 w987 w1034 w1058 w1098 w1115 w1127 w1148 w1170 w1189 w1204 w1226 w1243 w1264 w1279 w1324 w1338 w1357 w1370 w1389 w1403 w1427 w1449 w1461 w1492 w1550 w1575 w1594 w1619 w1637] -> w786
              tunnel: w785 -> [_ _ _ w884 _ _ _ _ _ _ _ _ _ _ _ _ _ _ _ _ _ _ _ _ _ _ _ _ _ _ _ _ _ _ _ _ _]
              tunnel: w784 -> [w810 w835 w871 _ _ _ _ _ w986 w1033 w1057 w1097 w1114 w1126 w1147 w1169 w1188 w1203 w1225 w1242 w1263 w1280 w1325 w1337 w1356 w1369 w1388 w1402 w1426 w1448 w1460 w1491 w1549 w1574 w1593 w1618 w1636]
              tunnel: [w810 w835 w871 _ _ _ _ _ w986 w1033 w1057 w1097 w1114 w1126 w1147 w1169 w1188 w1203 w1225 w1242 w1263 w1280 w1325 w1337 w1356 w1369 w1388 w1402 w1426 w1448 w1460 w1491 w1549 w1574 w1593 w1618 w1636] -> w783
              tunnel: w782 -> [_ _ _ _ w891 w923 w953 _ _ _ _ _ _ _ _ _ _ _ _ _ _ _ _ _ _ _ _ _ _ _ _ _ _ _ _ _ _]
              tunnel: w781 -> [_ _ _ _ _ _ _ _ w983 _ _ _ _ _ _ w1161 w1180 _ _ _ _ _ _ _ _ _ _ _ _ _ _ _ _ _ _ _ _]
              tunnel: w780 -> [_ _ _ _ _ _ _ _ _ _ _ _ _ _ _ _ _ _ _ _ _ _ _ _ _ _ _ _ _ _ _ _ _ _ _ _ w1630]
              frame "", Default {
              }
              frame "m0_0" {
                w827 = 2
                w829 = FALSE ("已勾选")
                n235 = property on="CAN Channel" class="Enum (严格)"() -> ("Value"=w825:enum16{"1", "2"})  [unwired: 2 in, 2 out]
                n236 = Set Menu Item Info(6:TRUE ("已勾选"), 7:"m0_0" ("项标识符"), 11:w841) -> (3:w840:refnum<k9>)  [unwired: 4 in, 1 out]
                n237 = Equal?(x=w825, y=enum16{"1", "2"}."2") -> (x = y?=w823:bool)
                n238 = case shown="真" w823 {
                  frame False {
                  }
                  frame True {
                    n239 = property on="CAN Channel" class="Enum (严格)"("Value"=enum16{"1", "2"}."1" ("CAN Channel")) -> ()  [unwired: 2 in, 2 out]
                  }
                }
                n240 = Set Menu Item Info(6:w829, 7:"m0_1" ("项标识符"), 11:w840) -> (3:w830:refnum<k9>)  [unwired: 4 in, 1 out]
                n241 = Set Menu Item Info(7:"m2_6_1" ("项标识符"), 9:w829, 11:w830) -> ()  [unwired: 4 in, 2 out]
                n242 = Set Menu Item Info(7:"m2_7_1" ("项标识符"), 9:w829, 11:w830) -> ()  [unwired: 4 in, 2 out]
                n243 = Set Menu Item Info(7:"m4_6_1" ("项标识符"), 9:w829, 11:w830) -> ()  [unwired: 4 in, 2 out]
                n244 = Set Menu Item Info(7:"m4_7_1" ("项标识符"), 9:w829, 11:w830) -> ()  [unwired: 4 in, 2 out]
                n245 = Open VI Reference(vi path=path "DeviceOP/ReciveThread.vi" ("VI路径")) -> (vi reference=w819:refnum<vi>, error out=w821:errorcluster)  [unwired: 5 in]
                n246 = property on="errcnt2" class="DigNum (严格)"("DisabledEnum"=w827) -> ()  [unwired: 2 in, 2 out]
                n247 = property on="Trate2" class="DigNum (严格)"("DisabledEnum"=w827) -> ()  [unwired: 2 in, 2 out]
                n248 = property on="Rrate2" class="DigNum (严格)"("DisabledEnum"=w827) -> ()  [unwired: 2 in, 2 out]
                n249 = invoke class="VI" method="Ctrl Val.Set"(reference=w819, error in=w821, "Control Name"="Enable2" ("控件名"), "Value"=FALSE) -> (reference out=w817:refnum<vi>, error out=w816:errorcluster)  [unwired: 1 in, 3 out]
                n250 = property on="CAN Channel" class="Enum (严格)"("Disabled Items []"=i32[] [1] ("禁用项[]")) -> ()  [unwired: 2 in, 2 out]
                n251 = Close Reference(reference=w817, error in (no error)=w816) -> ()  [unwired: 1 out]
                n252 = Bundle By Name(cluster=w828, "type"=u16 3 ("devtype")) -> (w838:T2)
              }
              frame "m0_1" {
                w857 = 2
                w858 = 0
                w865 = TRUE ("已勾选")
                n253 = Set Menu Item Info(6:FALSE ("已勾选"), 7:"m0_0" ("项标识符"), 11:w875) -> (3:w877:refnum<k9>)  [unwired: 4 in, 1 out]
                n254 = Unbundle By Name(w864) -> ("rateR2"=w863:bool, "rateT2"=w861:bool, "chk2"=w851:bool, "RcvE2"=w850:bool)
                n255 = Set Menu Item Info(6:w865, 7:"m0_1" ("项标识符"), 11:w877) -> (3:w866:refnum<k9>)  [unwired: 4 in, 1 out]
                n256 = Set Menu Item Info(7:"m2_6_1" ("项标识符"), 9:w865, 11:w866) -> ()  [unwired: 4 in, 2 out]
                n257 = Set Menu Item Info(7:"m2_7_1" ("项标识符"), 9:w865, 11:w866) -> ()  [unwired: 4 in, 2 out]
                n258 = Set Menu Item Info(7:"m4_6_1" ("项标识符"), 9:w865, 11:w866) -> ()  [unwired: 4 in, 2 out]
                n259 = Set Menu Item Info(7:"m4_7_1" ("项标识符"), 9:w865, 11:w866) -> ()  [unwired: 4 in, 2 out]
                n260 = Bundle By Name(cluster=w864, "type"=u16 4 ("devtype")) -> (w874:T2)
                n261 = Select(t=w858, s=w861, f=w857) -> (s? t:f=w860:i32)
                n262 = Select(t=w858, s=w863, f=w857) -> (s? t:f=w862:i32)
                n263 = Select(t=w858, s=w851, f=w857) -> (s? t:f=w859:i32)
                n264 = property on="Trate2" class="DigNum (严格)"("DisabledEnum"=w860) -> ()  [unwired: 2 in, 2 out]
                n265 = property on="errcnt2" class="DigNum (严格)"("DisabledEnum"=w859) -> ()  [unwired: 2 in, 2 out]
                n266 = property on="Rrate2" class="DigNum (严格)"("DisabledEnum"=w862) -> ()  [unwired: 2 in, 2 out]
                n267 = property on="CAN Channel" class="Enum (严格)"("Disabled Items []"=i32[] [] ("禁用项[]")) -> ()  [unwired: 2 in, 2 out]
                n268 = Open VI Reference(vi path=path "DeviceOP/ReciveThread.vi" ("VI路径")) -> (vi reference=w854:refnum<vi>, error out=w852:errorcluster)  [unwired: 5 in]
                n269 = invoke class="VI" method="Ctrl Val.Set"(reference=w854, error in=w852, "Control Name"="Enable2" ("控件名"), "Value"=w850) -> (reference out=w849:refnum<vi>, error out=w848:errorcluster)  [unwired: 1 in, 3 out]
                n270 = Close Reference(reference=w849, error in (no error)=w848) -> ()  [unwired: 1 out]
              }
              frame "m1_0" {
                n271 = Generate User Event(user event=w884, event data cluster=TRUE ("事件数据")) -> ()  [unwired: 1 in, 2 out]
              }
              frame "m1_1" {
                w890 = FALSE
                n272 = case shown="真" w895 {
                  tunnel: w894 -> [_ w899]
                  frame False {
                    n273 = call "TimeLmtDialog.vi"("Infoin"="设备已关闭！") -> ()  [unwired: 11 in]
                  }
                  frame True {
                    n274 = local read "DevIndex"() -> (w898:u32)
                    n275 = stacked-sequence {
                      tunnel: w899 -> [w901 w911]
                      tunnel: w898 -> [w900 w910]
                      frame #0 {
                        n276 = Equal?(x=w901, y=u16 4) -> (x = y?=w905:bool)
                        n277 = Select(t=2, s=w905, f=1) -> (s? t:f=w902:i32)
                        n278 = for {
                          N: w902 -> [_]
                          tunnel: w901 -> [w909]
                          tunnel: w900 -> [w908]
                          i -> [w907]
                          n279 = call "ResetCAN.vi"("CANInd"=w907, "DeciceInd"=w908, "DeviceType"=w909) -> ()  [unwired: 7 in, 2 out]
                        }
                      }
                      frame #1 {
                        n280 = call "CloseDevice.vi"("DeviceInd"=w910, "type"=w911) -> ("success"=w912:bool)  [unwired: 8 in, 1 out]
                        n281 = case shown="真" w912 {
                          frame False {
                            n282 = call "TimeLmtDialog.vi"("Infoin"="关闭失败！") -> ()  [unwired: 11 in]
                          }
                          frame True {
                            n283 = call "TimeLmtDialog.vi"("Infoin"="关闭成功！") -> ()  [unwired: 11 in]
                          }
                        }
                      }
                    }
                  }
                }
                n284 = global write "_USB_CAN_GLOBAL_.vi" "open"(FALSE ("open")) -> ()
                n285 = property class="VI"("Front Panel.Title"=w891) -> ()  [unwired: 2 in, 2 out]
              }
              frame "m1_3" {
                w922 = FALSE
                n286 = case shown="真" w926 {
                  tunnel: w925 -> [_ w929]
                  frame False {
                  }
                  frame True {
                    n287 = local read "DevIndex"() -> (w928:u32)
                    n288 = stacked-sequence {
                      tunnel: w929 -> [w931 w941]
                      tunnel: w928 -> [w930 w940]
                      frame #0 {
                        n289 = Equal?(x=w931, y=u16 4) -> (x = y?=w935:bool)
                        n290 = Select(t=2, s=w935, f=1) -> (s? t:f=w932:i32)
                        n291 = for {
                          N: w932 -> [_]
                          tunnel: w931 -> [w939]
                          tunnel: w930 -> [w938]
                          i -> [w937]
                          n292 = call "ResetCAN.vi"("CANInd"=w937, "DeciceInd"=w938, "DeviceType"=w939) -> ()  [unwired: 7 in, 2 out]
                        }
                      }
                      frame #1 {
                        n293 = call "CloseDevice.vi"("DeviceInd"=w940, "type"=w941) -> ("success"=w942:bool)  [unwired: 8 in, 1 out]
                        n294 = case shown="真" w942 {
                          frame False {
                            n295 = call "TimeLmtDialog.vi"("Infoin"="关闭失败！") -> ()  [unwired: 11 in]
                          }
                          frame True {
                            n296 = call "TimeLmtDialog.vi"("Infoin"="关闭成功！") -> ()  [unwired: 11 in]
                          }
                        }
                      }
                    }
                  }
                }
                n297 = global write "_USB_CAN_GLOBAL_.vi" "open"(FALSE ("open")) -> ()
                n298 = call "Global_Application Path.vi"() -> ("程序路径"=w918:path)  [unwired: 1 in]
                n299 = Build Path(base path=w918, name or relative path="波特率侦测.exe " ("command line")) -> (appended path=w916:path)
                n300 = Path To String(path=w916) -> (string=w915:string)
                n301 = call <vilib>:"System Exec.vi"("wait until completion? (T)"=FALSE, "command line"=w915) -> ("error out"=w919:errorcluster)  [unwired: 6 in, 3 out]
                n302 = call <vilib>:"Simple Error Handler.vi"("error in (no error)"=w919) -> ()  [unwired: 4 in, 5 out]
                n303 = property class="VI"("Front Panel.Title"=w923) -> ()  [unwired: 2 in, 2 out]
              }
              frame "m1_4" {
                w952 = FALSE
                n304 = case shown="真" w956 {
                  tunnel: w955 -> [_ w959]
                  frame False {
                  }
                  frame True {
                    n305 = local read "DevIndex"() -> (w958:u32)
                    n306 = stacked-sequence {
                      tunnel: w959 -> [w961 w971]
                      tunnel: w958 -> [w960 w970]
                      frame #0 {
                        n307 = Equal?(x=w961, y=u16 4) -> (x = y?=w965:bool)
                        n308 = Select(t=2, s=w965, f=1) -> (s? t:f=w962:i32)
                        n309 = for {
                          N: w962 -> [_]
                          tunnel: w961 -> [w969]
                          tunnel: w960 -> [w968]
                          i -> [w967]
                          n310 = call "ResetCAN.vi"("CANInd"=w967, "DeciceInd"=w968, "DeviceType"=w969) -> ()  [unwired: 7 in, 2 out]
                        }
                      }
                      frame #1 {
                        n311 = call "CloseDevice.vi"("DeviceInd"=w970, "type"=w971) -> ("success"=w972:bool)  [unwired: 8 in, 1 out]
                        n312 = case shown="真" w972 {
                          frame False {
                            n313 = call "TimeLmtDialog.vi"("Infoin"="关闭失败！") -> ()  [unwired: 11 in]
                          }
                          frame True {
                            n314 = call "TimeLmtDialog.vi"("Infoin"="关闭成功！") -> ()  [unwired: 11 in]
                          }
                        }
                      }
                    }
                  }
                }
                n315 = global write "_USB_CAN_GLOBAL_.vi" "open"(FALSE ("open")) -> ()
                n316 = call "Global_Application Path.vi"() -> ("程序路径"=w948:path)  [unwired: 1 in]
                n317 = Build Path(base path=w948, name or relative path="CANBridgeConfig.exe " ("command line")) -> (appended path=w946:path)
                n318 = Path To String(path=w946) -> (string=w945:string)
                n319 = call <vilib>:"System Exec.vi"("wait until completion? (T)"=FALSE, "command line"=w945) -> ("error out"=w949:errorcluster)  [unwired: 6 in, 3 out]
                n320 = call <vilib>:"Simple Error Handler.vi"("error in (no error)"=w949) -> ()  [unwired: 4 in, 5 out]
                n321 = property class="VI"("Front Panel.Title"=w953) -> ()  [unwired: 2 in, 2 out]
              }
              frame "m1_2" {
                n322 = global read "_USB_CAN_GLOBAL_.vi" "open"() -> (w976:bool)
                n323 = case shown="假" w976 {
                  tunnel: w975 -> [_ w982]
                  frame False {
                    n324 = call "TimeLmtDialog.vi"("Infoin"="CAN设备未打开！") -> ()  [unwired: 11 in]
                  }
                  frame True {
                    n325 = local read "DevIndex"() -> (w981:u32)
                    n326 = call "CanStatusShow.vi"("DevIndex"=w981, "DevType"=w982) -> ()  [unwired: 10 in]
                  }
                }
              }
              frame "m2_0" {
                n327 = global read "_USB_CAN_GLOBAL_.vi" "open"() -> (w985:bool)
                n328 = case shown="真" w985 {
                  selector: w985 -> [_ w998]
                  tunnel: w990 -> [w993 w997]
                  tunnel: [w993 w996] -> w989
                  tunnel: w988 -> [_ w999]
                  tunnel: w984 -> [_ w995]
                  tunnel: w983 -> [_ w994]
                  frame False {
                    n329 = call "TimeLmtDialog.vi"("Infoin"="CAN设备未打开！") -> ()  [unwired: 11 in]
                  }
                  frame True {
                    n330 = stacked-sequence {
                      tunnel: w999 -> [_ w1016 _]
                      tunnel: w998 -> [_ w1015 _]
                      tunnel: w997 -> [_ w1012 _]
                      tunnel: [_ w1011 _] -> w996
                      tunnel: w995 -> [_ _ w1027]
                      tunnel: w994 -> [w1003 _ _]
                      frame #0 {
                        w1001 = FALSE
                        n331 = invoke class="VI" method="Ctrl Val.Set"(reference=w1003, "Control Name"="Enable" ("控件名"), "Value"=w1001) -> ()  [unwired: 2 in, 5 out]
                        n332 = Open VI Reference(vi path=path "DeviceOP/ReciveThread.vi" ("VI路径")) -> (vi reference=w1004:refnum<vi>, error out=w1005:errorcluster)  [unwired: 5 in]
                        n333 = invoke class="VI" method="Ctrl Val.Set"(reference=w1004, error in=w1005, "Control Name"="Enable1" ("控件名"), "Value"=w1001) -> (reference out=w1008:refnum<vi>, error out=w1009:errorcluster)  [unwired: 1 in, 3 out]
                        n334 = Not(x=w1001) -> (.not. x?=w1000:bool)
                        n335 = invoke class="VI" method="Ctrl Val.Set"(reference=w1008, error in=w1009, "Control Name"="Enable2" ("控件名"), "Value"=w1001) -> ()  [unwired: 1 in, 5 out]
                        n336 = property on="send stop" class="Bool (严格)"("Val(Sgnl)"=w1000) -> ()  [unwired: 2 in, 2 out]
                      }
                      frame #1 {
                        n337 = local read "DevIndex"() -> (w1017:u32)
                        n338 = call "CAN-SET.vi"("DevIndex"=w1017, "open?"=w1015, "type"=w1016) -> ("success"=w1014:bool, "Param out"=w1013:T5[])  [unwired: 7 in]
                        n339 = Select(t=w1013, s=w1014, f=w1012) -> (s? t:f=w1011:T5[])
                      }
                      frame #2 {
                        n340 = Unbundle By Name(w1027) -> ("RcvE1"=w1026:bool, "RcvE2"=w1025:bool)
                        n341 = Open VI Reference(vi path=path "DeviceOP/ReciveThread.vi" ("VI路径")) -> (vi reference=w1018:refnum<vi>, error out=w1019:errorcluster)  [unwired: 5 in]
                        n342 = invoke class="VI" method="Ctrl Val.Set"(reference=w1018, error in=w1019, "Control Name"="Enable1" ("控件名"), "Value"=w1026) -> (reference out=w1022:refnum<vi>, error out=w1023:errorcluster)  [unwired: 1 in, 3 out]
                        n343 = invoke class="VI" method="Ctrl Val.Set"(reference=w1022, error in=w1023, "Control Name"="Enable2" ("控件名"), "Value"=w1025) -> ()  [unwired: 1 in, 5 out]
                      }
                    }
                  }
                }
              }
              frame "m2_1" {
                n344 = Two Button Dialog(message="是否确定恢复出厂设置？" ("消息")) -> (T button?=w1029:bool)  [unwired: 2 in]
                n345 = case shown="真" w1029 {
                  tunnel: w1031 -> [_ w1044]
                  tunnel: w1030 -> [_ _]
                  frame False {
                  }
                  frame True {
                    n346 = local read "DevIndex"() -> (w1045:u32)
                    n347 = Equal?(x=u16 4, y=w1044) -> (x = y?=w1042:bool)
                    n348 = Select(t=2, s=w1042, f=1) -> (s? t:f=w1039:i32)
                    n349 = for {
                      N: w1039 -> [_]
                      tunnel: w1045 -> [w1051]
                      tunnel: w1044 -> [w1050]
                      tunnel: [w1048] -> w1038 mode=indexing
                      i -> [w1049]
                      n350 = call "ResumeConfig.vi"("CANInd"=w1049, "DeciceInd"=w1051, "DeviceType"=w1050) -> ("Success"=w1052:bool)  [unwired: 7 in, 1 out]
                      n351 = case shown="真" w1052 {
                        tunnel: w1050 -> [_ w1056]
                        tunnel: w1051 -> [_ w1055]
                        tunnel: [_ w1054] -> w1048
                        tunnel: w1049 -> [_ w1053]
                        frame False {
                        }
                        frame True {
                          n352 = call "StartCAN.vi"("CANInd"=w1053, "DeciceInd"=w1055, "DeviceType"=w1056) -> ("Valid"=w1054:bool)  [unwired: 7 in, 1 out]
                        }
                      }
                    }
                    n353 = And Array Elements(Boolean array=w1038) -> (logical AND=w1037:bool)
                    n354 = case shown="真" w1037 {
                      frame False {
                        n355 = call "TimeLmtDialog.vi"("Infoin"="操作失败！") -> ()  [unwired: 11 in]
                      }
                      frame True {
                        n356 = call "TimeLmtDialog.vi"("Infoin"="恢复成功！") -> ()  [unwired: 11 in]
                      }
                    }
                  }
                }
              }
              frame "m2_2" {
                n357 = case shown="真" w1060 {
                  tunnel: w1059 -> [_ w1065]
                  frame False {
                    n358 = call "TimeLmtDialog.vi"("Infoin"="请先打开USB-CAN设备，再进行此操作！") -> ()  [unwired: 11 in]
                  }
                  frame True {
                    n359 = local read "DevIndex"() -> (w1064:u32)
                    n360 = call "ReadBoardInfo.vi"("DeviceInd"=w1064, "DeviceType"=w1065) -> ("VCI_BOARD_INFO"=w1066:T6, "success"=w1067:bool)  [unwired: 8 in]
                    n361 = case shown="真" w1067 {
                      tunnel: w1066 -> [_ _]
                      tunnel: w1065 -> [_ w1071]
                      tunnel: w1064 -> [_ w1070]
                      tunnel: w1064 -> [_ w1069]
                      frame False {
                        n362 = call "TimeLmtDialog.vi"("Infoin"="获取设备信息失败！") -> ()  [unwired: 11 in]
                      }
                      frame True {
                        n363 = call "_USB_CAN_BI_.vi"() -> ("change?"=w1073:bool, "BOARD_INFO out"=w1072:T7)  [unwired: 10 in]
                        n364 = case shown="真" w1073 {
                          tunnel: w1072 -> [_ w1078]
                          tunnel: w1071 -> [_ w1075]
                          tunnel: w1070 -> [_ w1077]
                          tunnel: w1069 -> [_ w1074]
                          frame False {
                          }
                          frame True {
                            n365 = call "WriteBoardInfo.vi"("BOARD_INFO"=w1078, "DeviceInd"=w1077, "DeviceType"=w1075) -> ("success"=w1076:bool)  [unwired: 8 in]
                            n366 = case shown="真" w1076 {
                              tunnel: w1075 -> [_ w1082]
                              tunnel: w1074 -> [_ w1081]
                              frame False {
                                n367 = call "TimeLmtDialog.vi"("Infoin"="修改失败！") -> ()  [unwired: 11 in]
                              }
                              frame True {
                                n368 = call "DeviceReset.vi"("DeviceInd"=w1081, "DeviceType"=w1082) -> ("Success"=w1080:bool)  [unwired: 9 in]
                                n369 = case shown="真" w1080 {
                                frame False {
                                n370 = call "TimeLmtDialog.vi"("Infoin"="修改完成，但设备重置时出错！") -> ()  [unwired: 11 in]
                                }
                                frame True {
                                n371 = call "TimeLmtDialog.vi"("Infoin"="修改成功！") -> ()  [unwired: 11 in]
                                }
                                }
                              }
                            }
                          }
                        }
                      }
                    }
                  }
                }
              }
              frame "m2_3" {
                n372 = Unbundle By Name(w1091) -> ("scantime"=w1096:u16)
                n373 = Open VI Reference(vi path=path "DeviceOP/ReciveThread.vi" ("VI路径")) -> (vi reference=w1087:refnum<vi>, error out=w1086:errorcluster)  [unwired: 5 in]
                n374 = call "Scan time Input.vi"("In"=w1096) -> ("out"=w1085:u32)  [unwired: 10 in]
                n375 = Bundle By Name(cluster=w1091, "scantime"=w1085) -> (w1090:T2)
                n376 = invoke class="VI" method="Ctrl Val.Set"(reference=w1087, error in=w1086, "Control Name"="Scan time" ("控件名"), "Value"=w1085) -> ()  [unwired: 1 in, 5 out]
                n377 = Format Into String(format string="接收扫描时间(%dms)" ("格式字符串"), w1085) -> (resulting string=w1092:string)  [unwired: 2 in, 1 out]
                n378 = Set Menu Item Info(7:w1093, 10:w1092, 11:w1094) -> ()  [unwired: 4 in, 2 out]
              }
              frame "m2_9" {
                n379 = Unbundle By Name(w1111) -> ("RcvLen"=w1109:i16)
                n380 = Open VI Reference(vi path=path "DeviceOP/ReciveThread.vi" ("VI路径")) -> (vi reference=w1104:refnum<vi>, error out=w1103:errorcluster)  [unwired: 5 in]
                n381 = call "Scan time Input.vi"("In"=w1109) -> ("out"=w1102:u32)  [unwired: 10 in]
                n382 = Bundle By Name(cluster=w1111, "RcvLen"=w1102) -> (w1110:T2)
                n383 = invoke class="VI" method="Ctrl Val.Set"(reference=w1104, error in=w1103, "Control Name"="RcvLen" ("控件名"), "Value"=w1102) -> ()  [unwired: 1 in, 5 out]
                n384 = Format Into String(format string="每次接收帧数(%d)" ("格式字符串"), w1102) -> (resulting string=w1107:string)  [unwired: 2 in, 1 out]
                n385 = Set Menu Item Info(7:w1112, 10:w1107, 11:w1113) -> ()  [unwired: 4 in, 2 out]
              }
              frame "m2_4_0" {
                n386 = Get Menu Item Info(7:w1134, 11:w1135) -> (3:w1136:refnum<k9>, 4:w1119:bool)  [unwired: 1 in, 5 out]
                n387 = Not(x=w1119) -> (.not. x?=w1125:bool)
                n388 = Set Menu Item Info(6:w1125, 7:w1134, 11:w1136) -> (3:w1121:refnum<k9>)  [unwired: 4 in, 1 out]
                n389 = Set Menu Item Info(6:w1119, 7:"m2_4_1" ("项标识符"), 11:w1121) -> ()  [unwired: 4 in, 2 out]
                n390 = Open VI Reference(vi path=path "DeviceOP/ReciveThread.vi" ("VI路径")) -> (vi reference=w1130:refnum<vi>, error out=w1128:errorcluster)  [unwired: 5 in]
                n391 = Select(t=u16 1 ("Rfun"), s=w1125, f=u16 2 ("Rfun")) -> (s? t:f=w1122:u16)
                n392 = invoke class="VI" method="Ctrl Val.Set"(reference=w1130, error in=w1128, "Control Name"="RFun" ("控件名"), "Value"=w1122) -> ()  [unwired: 1 in, 5 out]
                n393 = Bundle By Name(cluster=w1132, "Rfun"=w1122) -> (w1133:T2)
              }
              frame "m2_4_1" {
                n394 = Get Menu Item Info(7:w1155, 11:w1156) -> (3:w1157:refnum<k9>, 4:w1140:bool)  [unwired: 1 in, 5 out]
                n395 = Not(x=w1140) -> (.not. x?=w1146:bool)
                n396 = Set Menu Item Info(6:w1146, 7:w1155, 11:w1157) -> (3:w1142:refnum<k9>)  [unwired: 4 in, 1 out]
                n397 = Set Menu Item Info(6:w1140, 7:"m2_4_0" ("项标识符"), 11:w1142) -> ()  [unwired: 4 in, 2 out]
                n398 = Open VI Reference(vi path=path "DeviceOP/ReciveThread.vi" ("VI路径")) -> (vi reference=w1151:refnum<vi>, error out=w1149:errorcluster)  [unwired: 5 in]
                n399 = Select(t=u16 2 ("Rfun"), s=w1146, f=u16 1 ("Rfun")) -> (s? t:f=w1143:u16)
                n400 = invoke class="VI" method="Ctrl Val.Set"(reference=w1151, error in=w1149, "Control Name"="RFun" ("控件名"), "Value"=w1143) -> ()  [unwired: 1 in, 5 out]
                n401 = Bundle By Name(cluster=w1153, "Rfun"=w1143) -> (w1154:T2)
              }
              frame "m2_5_0" {
                n402 = Get Menu Item Info(7:w1174, 11:w1175) -> (3:w1176:refnum<k9>, 4:w1162:bool)  [unwired: 1 in, 5 out]
                n403 = Not(x=w1162) -> (.not. x?=w1168:bool)
                n404 = Set Menu Item Info(6:w1168, 7:w1174, 11:w1176) -> (3:w1164:refnum<k9>)  [unwired: 4 in, 1 out]
                n405 = Set Menu Item Info(6:w1162, 7:"m2_5_1" ("项标识符"), 11:w1164) -> ()  [unwired: 4 in, 2 out]
                n406 = Select(t=u16 1 ("Rfun"), s=w1168, f=u16 2 ("Rfun")) -> (s? t:f=w1165:u16)
                n407 = invoke class="VI" method="Ctrl Val.Set"(reference=w1161, "Control Name"="TFun" ("控件名"), "Value"=w1165) -> ()  [unwired: 2 in, 5 out]
                n408 = Bundle By Name(cluster=w1172, "Tfun"=w1165) -> (w1173:T2)
              }
              frame "m2_5_1" {
                n409 = Get Menu Item Info(7:w1193, 11:w1194) -> (3:w1195:refnum<k9>, 4:w1181:bool)  [unwired: 1 in, 5 out]
                n410 = Not(x=w1181) -> (.not. x?=w1187:bool)
                n411 = Set Menu Item Info(6:w1187, 7:w1193, 11:w1195) -> (3:w1183:refnum<k9>)  [unwired: 4 in, 1 out]
                n412 = Set Menu Item Info(6:w1181, 7:"m2_5_0" ("项标识符"), 11:w1183) -> ()  [unwired: 4 in, 2 out]
                n413 = Select(t=u16 2 ("Rfun"), s=w1187, f=u16 1 ("Rfun")) -> (s? t:f=w1184:u16)
                n414 = invoke class="VI" method="Ctrl Val.Set"(reference=w1180, "Control Name"="TFun" ("控件名"), "Value"=w1184) -> ()  [unwired: 2 in, 5 out]
                n415 = Bundle By Name(cluster=w1191, "Tfun"=w1184) -> (w1192:T2)
              }
              frame "m2_6_0" {
                n416 = Get Menu Item Info(7:w1209, 11:w1210) -> (3:w1212:refnum<k9>, 4:w1211:bool)  [unwired: 1 in, 5 out]
                n417 = Not(x=w1211) -> (.not. x?=w1202:bool)
                n418 = Set Menu Item Info(6:w1202, 7:w1209, 11:w1212) -> ()  [unwired: 4 in, 2 out]
                n419 = invoke class="VI" method="Ctrl Val.Set"(reference=w1208, "Control Name"="check1" ("控件名"), "Value"=w1202) -> ()  [unwired: 2 in, 5 out]
                n420 = Select(t=T4."Enabled" ("禁用"), s=w1202, f=T4."Disabled and Grayed Out" ("禁用")) -> (s? t:f=w1199:T4)
                n421 = Bundle By Name(cluster=w1205, "chk1"=w1202) -> (w1206:T2)
                n422 = property on="errcnt1" class="DigNum (严格)"("DisabledEnum"=w1199) -> ()  [unwired: 2 in, 2 out]
              }
              frame "m2_6_1" {
                n423 = Get Menu Item Info(7:w1230, 11:w1231) -> (3:w1233:refnum<k9>, 4:w1232:bool)  [unwired: 1 in, 5 out]
                n424 = Not(x=w1232) -> (.not. x?=w1217:bool)
                n425 = Set Menu Item Info(6:w1217, 7:w1230, 11:w1233) -> ()  [unwired: 4 in, 2 out]
                n426 = Unbundle By Name(w1221) -> ("type"=w1220:u16)
                n427 = Equal?(x=u16 4, y=w1220) -> (x = y?=w1218:bool)
                n428 = And(x=w1218, y=w1217) -> (x .and. y?=w1216:bool)
                n429 = Bundle By Name(cluster=w1221, "chk2"=w1217) -> (w1227:T2)
                n430 = invoke class="VI" method="Ctrl Val.Set"(reference=w1229, "Control Name"="check2" ("控件名"), "Value"=w1216) -> ()  [unwired: 2 in, 5 out]
                n431 = Select(t=T4."Enabled" ("禁用"), s=w1216, f=T4."Disabled and Grayed Out" ("禁用")) -> (s? t:f=w1222:T4)
                n432 = property on="errcnt2" class="DigNum (严格)"("DisabledEnum"=w1222) -> ()  [unwired: 2 in, 2 out]
              }
              frame "m2_7_0" {
                n433 = Get Menu Item Info(7:w1246, 11:w1247) -> (3:w1249:refnum<k9>, 4:w1248:bool)  [unwired: 1 in, 5 out]
                n434 = Not(x=w1248) -> (.not. x?=w1237:bool)
                n435 = Set Menu Item Info(6:w1237, 7:w1246, 11:w1249) -> ()  [unwired: 4 in, 2 out]
                n436 = Open VI Reference(vi path=path "DeviceOP/ReciveThread.vi" ("VI路径")) -> (vi reference=w1240:refnum<vi>, error out=w1238:errorcluster)  [unwired: 5 in]
                n437 = invoke class="VI" method="Ctrl Val.Set"(reference=w1240, error in=w1238, "Control Name"="Enable1" ("控件名"), "Value"=w1237) -> ()  [unwired: 1 in, 5 out]
                n438 = Bundle By Name(cluster=w1244, "RcvE1"=w1237) -> (w1245:T2)
              }
              frame "m2_7_1" {
                n439 = Get Menu Item Info(7:w1266, 11:w1267) -> (3:w1269:refnum<k9>, 4:w1268:bool)  [unwired: 1 in, 5 out]
                n440 = Not(x=w1268) -> (.not. x?=w1254:bool)
                n441 = Set Menu Item Info(6:w1254, 7:w1266, 11:w1269) -> ()  [unwired: 4 in, 2 out]
                n442 = Unbundle By Name(w1255) -> ("type"=w1258:u16)
                n443 = Open VI Reference(vi path=path "DeviceOP/ReciveThread.vi" ("VI路径")) -> (vi reference=w1261:refnum<vi>, error out=w1259:errorcluster)  [unwired: 5 in]
                n444 = Equal?(x=u16 4, y=w1258) -> (x = y?=w1256:bool)
                n445 = And(x=w1256, y=w1254) -> (x .and. y?=w1253:bool)
                n446 = invoke class="VI" method="Ctrl Val.Set"(reference=w1261, error in=w1259, "Control Name"="Enable2" ("控件名"), "Value"=w1253) -> ()  [unwired: 1 in, 5 out]
                n447 = Bundle By Name(cluster=w1255, "RcvE2"=w1253) -> (w1265:T2)
              }
              frame "m2_8" {
                # "恢复出厂设置（软件参数重置）"
                n448 = Two Button Dialog(message="本操作将重置软件参数至初始状态。\n重置后将导致当前软件界面设置、CAN配置参数等丢失！\n重置后，重启本软件生效，是否确定重置？" ("消息")) -> (T button?=w1273:bool)  [unwired: 2 in]
                n449 = case shown="真" w1273 {
                  tunnel: w1275 -> [_ w1281]
                  frame False {
                  }
                  frame True {
                    n450 = stacked-sequence {
                      tunnel: w1281 -> [_ _ w1303 _ _]
                      frame #0 {
                        n451 = call "Global_Application Path.vi"() -> ("程序路径"=w1284:path)  [unwired: 1 in]
                        n452 = Build Path(base path=w1284, name or relative path="usb_can.ini" ("名称或相对路径")) -> (appended path=w1283:path)
                        n453 = Delete(path (use dialog)=w1283) -> (error out=w1282:errorcluster)  [unwired: 4 in, 2 out]
                        n454 = call <vilib>:"Clear Errors.vi"("error in (no error)"=w1282) -> ()  [unwired: 6 in, 1 out]
                      }
                      frame #1 {
                        n455 = property class="VI"() -> ("Name"=w1292:string)  [unwired: 2 in, 2 out]
                        n456 = call "Global_Application Path.vi"() -> ("程序路径"=w1289:path)  [unwired: 1 in]
                        n457 = String To Byte Array(string=w1292) -> (unsigned byte array=w1291:u8[])
                        n458 = for {
                          N: 4 -> [_]
                          tunnel: w1291 -> [w1301] mode=indexing
                          shift-right: [w1298] -> w1293
                          shift-left: "" -> [w1299]
                          n459 = Format Into String(format string="%02x" ("格式字符串"), initial string=w1299, w1301) -> (resulting string=w1298:string)  [unwired: 1 in, 1 out]
                        }
                        n460 = String Subset(string=w1293, length (rest)=16 ("长度（剩余）")) -> (substring=w1295:string)  [unwired: 1 in]
                        n461 = Concatenate Strings(w1295, ".uis" ("字符串")) -> (w1288:string)
                        n462 = Build Path(base path=w1289, name or relative path=w1288) -> (appended path=w1287:path)
                        n463 = Delete(path (use dialog)=w1287) -> (error out=w1286:errorcluster)  [unwired: 4 in, 2 out]
                        n464 = call <vilib>:"Clear Errors.vi"("error in (no error)"=w1286) -> ()  [unwired: 6 in, 1 out]
                      }
                      frame #2 {
                        n465 = local read "DevIndex"() -> (w1302:u32)
                        n466 = call "CloseDevice.vi"("DeviceInd"=w1302, "type"=w1303) -> ()  [unwired: 8 in, 2 out]
                      }
                      frame #3 {
                        n467 = call "Global_Application Path.vi"() -> ("程序路径"=w1310:path)  [unwired: 1 in]
                        n468 = call "Global_Application Path.vi"("Use ExeFilePath"=TRUE) -> ("程序路径"=w1309:path)
                        n469 = Path To String(path=w1309) -> (string=w1307:string)
                        n470 = Concatenate Strings("reboot.exe -- run \"" ("command line"), w1307, "\" w:4000 \"t:USB_CAN Tool -- Reboot\"" ("字符串")) -> (w1306:string)
                        n471 = call <vilib>:"System Exec.vi"("wait until completion? (T)"=FALSE, "working directory"=w1310, "command line"=w1306) -> ("error out"=w1311:errorcluster)  [unwired: 5 in, 3 out]
                        n472 = call <vilib>:"Clear Errors.vi"("error in (no error)"=w1311) -> ()  [unwired: 6 in, 1 out]
                      }
                      frame #4 {
                        n473 = control-ref of="本VI"() -> (w1313:refnum<vi>)
                        n474 = call "Exit.vi"("VI引用"=w1313) -> ()  [unwired: 10 in, 1 out]
                      }
                    }
                  }
                }
              }
              frame "m3_0" {
                n475 = Equal?(x=w1314, y=u16 4) -> (x = y?=w1318:bool)
                n476 = Select(t=2, s=w1318, f=1) -> (s? t:f=w1315:i32)
                n477 = for {
                  N: w1315 -> [_]
                  tunnel: w1314 -> [w1333]
                  tunnel: [w1331] -> w1323 mode=indexing
                  tunnel: [w1330] -> w1320 mode=indexing
                  i -> [w1328]
                  w1329 = u32 15 items=["REFTYPE_MODE"=0, "REFTYPE_FILTER"=1, "REFTYPE_ACR0"=2, "REFTYPE_AMR0"=6, "REFTYPE_kCANBAUD"=10, "REFTYPE_CANRX_EN"=13, "REFTYPE_UARTBAUD"=14, "REFTYPE_ALL"=15] ("RefType")
                  n478 = local read "DevIndex"() -> (w1332:u32)
                  n479 = call "GetReference2.vi"("DeviceType"=w1333, "DeviceInd"=w1332, "CANInd"=w1328, "RefType"=w1329) -> ("Success"=w1331:bool, "Param"=w1330:T5)  [unwired: 9 in, 1 out]
                }
                n480 = And Array Elements(Boolean array=w1323) -> (logical AND=w1322:bool)
                n481 = case shown="真" w1322 {
                  tunnel: w1320 -> [_ w1336]
                  tunnel: w1314 -> [_ w1335]
                  frame False {
                    n482 = call "TimeLmtDialog.vi"("Infoin"="获取失败！") -> ()  [unwired: 11 in]
                  }
                  frame True {
                    n483 = call "CAN_ParamShow.vi"("DevType"=w1335, "param"=w1336) -> ()  [unwired: 10 in]
                  }
                }
              }
              frame "m3_1" {
                n484 = case shown="真" w1340 {
                  tunnel: w1339 -> [_ w1347]
                  frame False {
                    n485 = call "TimeLmtDialog.vi"("Infoin"="请先打开USB-CAN设备，再进行此操作！") -> ()  [unwired: 11 in]
                  }
                  frame True {
                    n486 = local read "DevIndex"() -> (w1346:u32)
                    n487 = call "ReadBoardInfo.vi"("DeviceInd"=w1346, "DeviceType"=w1347) -> ("VCI_BOARD_INFO"=w1344:T6, "success"=w1345:bool)  [unwired: 8 in]
                    n488 = case shown="真" w1345 {
                      tunnel: w1344 -> [_ w1349]
                      frame False {
                        n489 = call "TimeLmtDialog.vi"("Infoin"="读取失败！") -> ()  [unwired: 11 in]
                      }
                      frame True {
                        n490 = call "_USB_CAN_BOARD_INFO_.vi"("VCI_BOARD_INFO"=w1349) -> ()  [unwired: 11 in]
                      }
                    }
                  }
                }
              }
              frame "m4_0" {
                n491 = Get Menu Item Info(7:w1363, 11:w1365) -> (3:w1364:refnum<k9>, 4:w1362:bool)  [unwired: 1 in, 5 out]
                n492 = Not(x=w1362) -> (.not. x?=w1351:bool)
                n493 = Set Menu Item Info(6:w1351, 7:w1363, 11:w1364) -> (3:w1352:refnum<k9>)  [unwired: 4 in, 1 out]
                n494 = invoke class="VI" method="Ctrl Val.Set"(reference=w1361, "Control Name"="highspd" ("控件名"), "Value"=w1351) -> ()  [unwired: 2 in, 5 out]
                n495 = Not(x=w1351) -> (.not. x?=w1350:bool)
                n496 = Set Menu Item Info(7:"m4_1" ("项标识符"), 9:w1350, 11:w1352) -> (3:w1355:refnum<k9>)  [unwired: 4 in, 1 out]
                n497 = Set Menu Item Info(7:"m4_2" ("项标识符"), 9:w1350, 11:w1355) -> ()  [unwired: 4 in, 2 out]
                n498 = Bundle By Name(cluster=w1359, "highspd"=w1351) -> (w1358:T2)
              }
              frame "m4_1" {
                n499 = Get Menu Item Info(7:w1377, 11:w1379) -> (3:w1378:refnum<k9>, 4:w1376:bool)  [unwired: 1 in, 5 out]
                n500 = Not(x=w1376) -> (.not. x?=w1373:bool)
                n501 = Set Menu Item Info(6:w1373, 7:w1377, 11:w1378) -> ()  [unwired: 4 in, 2 out]
                n502 = invoke class="VI" method="Ctrl Val.Set"(reference=w1375, "Control Name"="disp" ("控件名"), "Value"=w1373) -> ()  [unwired: 2 in, 5 out]
                n503 = Bundle By Name(cluster=w1372, "disp"=w1373) -> (w1371:T2)
              }
              frame "m4_2" {
                n504 = Get Menu Item Info(7:w1395, 11:w1397) -> (3:w1396:refnum<k9>, 4:w1394:bool)  [unwired: 1 in, 5 out]
                n505 = Not(x=w1394) -> (.not. x?=w1383:bool)
                n506 = Set Menu Item Info(6:w1383, 7:w1395, 11:w1396) -> ()  [unwired: 4 in, 2 out]
                n507 = invoke class="VI" method="Ctrl Val.Set"(reference=w1393, "Control Name"="save" ("控件名"), "Value"=w1383) -> (reference out=w1386:refnum<vi>, error out=w1385:errorcluster)  [unwired: 2 in, 3 out]
                n508 = Bundle By Name(cluster=w1391, "save"=w1383) -> (w1390:T2)
                n509 = invoke class="VI" method="Ctrl Val.Set"(reference=w1386, error in=w1385, "Control Name"="sPth_Sel" ("控件名"), "Value"=w1383) -> ()  [unwired: 1 in, 5 out]
                n510 = property on="path" class="Path"("Value"=path "" ("path")) -> ()  [unwired: 2 in, 2 out]
              }
              frame "m4_3" {
                n511 = Get Menu Item Info(7:w1407, 11:w1409) -> (3:w1408:refnum<k9>, 4:w1406:bool)  [unwired: 1 in, 5 out]
                n512 = Not(x=w1406) -> (.not. x?=w1401:bool)
                n513 = Set Menu Item Info(6:w1401, 7:w1407, 11:w1408) -> ()  [unwired: 4 in, 2 out]
                n514 = global write "_USB_CAN_GLOBAL_.vi" "Disp-HL"(w1401) -> ()
                n515 = Bundle By Name(cluster=w1405, "hl"=w1401) -> (w1404:T2)
              }
              frame "m4_8_0" {
                n516 = Get Menu Item Info(7:w1430, 11:w1431) -> (3:w1425:refnum<k9>, 4:w1423:bool)  [unwired: 1 in, 5 out]
                n517 = Set Menu Item Info(6:w1423, 7:"m4_8_1" ("项标识符"), 11:w1425) -> (3:w1422:refnum<k9>)  [unwired: 4 in, 1 out]
                n518 = Not(x=w1423) -> (.not. x?=w1421:bool)
                n519 = Set Menu Item Info(6:w1421, 7:w1430, 11:w1422) -> ()  [unwired: 4 in, 2 out]
                n520 = Select(t=enum16{"原始值", "实际值"}."原始值" ("TSFormat"), s=w1421, f=enum16{"原始值", "实际值"}."实际值" ("TSFormat")) -> (s? t:f=w1417:enum16{"原始值", "实际值"})
                n521 = invoke class="VI" method="Ctrl Val.Set"(reference=w1418, "Control Name"="TSFormat" ("控件名"), "Value"=w1417) -> (reference out=w1413:refnum<vi>)  [unwired: 2 in, 4 out]
                n522 = Bundle By Name(cluster=w1429, "TSFormat"=w1417) -> (w1428:T2)
                n523 = invoke class="VI" method="Ctrl Val.Set"(reference=w1413, "Control Name"="ForceUpt" ("控件名"), "Value"=TRUE) -> ()  [unwired: 2 in, 5 out]
              }
              frame "m4_8_1" {
                n524 = Get Menu Item Info(7:w1452, 11:w1453) -> (3:w1447:refnum<k9>, 4:w1445:bool)  [unwired: 1 in, 5 out]
                n525 = Set Menu Item Info(6:w1445, 7:"m4_8_0" ("项标识符"), 11:w1447) -> (3:w1444:refnum<k9>)  [unwired: 4 in, 1 out]
                n526 = Not(x=w1445) -> (.not. x?=w1443:bool)
                n527 = Set Menu Item Info(6:w1443, 7:w1452, 11:w1444) -> ()  [unwired: 4 in, 2 out]
                n528 = Select(t=enum16{"原始值", "实际值"}."实际值" ("TSFormat"), s=w1443, f=enum16{"原始值", "实际值"}."原始值" ("TSFormat")) -> (s? t:f=w1439:enum16{"原始值", "实际值"})
                n529 = invoke class="VI" method="Ctrl Val.Set"(reference=w1440, "Control Name"="TSFormat" ("控件名"), "Value"=w1439) -> (reference out=w1435:refnum<vi>)  [unwired: 2 in, 4 out]
                n530 = Bundle By Name(cluster=w1451, "TSFormat"=w1439) -> (w1450:T2)
                n531 = invoke class="VI" method="Ctrl Val.Set"(reference=w1435, "Control Name"="ForceUpt" ("控件名"), "Value"=TRUE) -> ()  [unwired: 2 in, 5 out]
              }
              frame "m4_4" {
                n532 = Get Menu Item Info(7:w1468, 11:w1470) -> (3:w1469:refnum<k9>, 4:w1467:bool)  [unwired: 1 in, 5 out]
                n533 = Not(x=w1467) -> (.not. x?=w1463:bool)
                n534 = Set Menu Item Info(6:w1463, 7:w1468, 11:w1469) -> ()  [unwired: 4 in, 2 out]
                n535 = invoke class="VI" method="Ctrl Val.Set"(reference=w1466, "Control Name"="ID合并" ("控件名"), "Value"=w1463) -> (reference out=w1459:refnum<vi>)  [unwired: 2 in, 4 out]
                n536 = Bundle By Name(cluster=w1464, "ID合并"=w1463) -> (w1462:T2)
                n537 = invoke class="VI" method="Ctrl Val.Set"(reference=w1459, "Control Name"="ForceUpt" ("控件名"), "Value"=TRUE) -> ()  [unwired: 2 in, 5 out]
              }
              frame "m4_5_0", "m4_5_1", "m4_5_2", "m4_5_3" {
                n538 = case shown="\"m4_5_0\"" w1485 {
                  tunnel: [TRUE FALSE FALSE FALSE] -> w1490
                  tunnel: [FALSE TRUE FALSE FALSE] -> w1489
                  tunnel: [FALSE FALSE TRUE FALSE] -> w1488
                  tunnel: [FALSE FALSE FALSE TRUE] -> w1487
                  tunnel: [enum16{"hex", "dec", "oct", "bin"}."hex" ("format") enum16{"hex", "dec", "oct", "bin"}."dec" ("format") enum16{"hex", "dec", "oct", "bin"}."oct" ("format") enum16{"hex", "dec", "oct", "bin"}."bin" ("format")] -> w1474
                  frame "m4_5_3", Default {
                  }
                  frame "m4_5_2" {
                  }
                  frame "m4_5_1" {
                  }
                  frame "m4_5_0" {
                  }
                }
                n539 = invoke class="VI" method="Ctrl Val.Set"(reference=w1483, "Control Name"="format" ("控件名"), "Value"=w1474) -> (reference out=w1478:refnum<vi>)  [unwired: 2 in, 4 out]
                n540 = for {
                  shift-right: [w1503] -> w1481
                  shift-left: w1486 -> [w1504]
                  tunnel: string[] ["m4_5_3", "m4_5_2", "m4_5_1", "m4_5_0"] -> [w1502] mode=indexing
                  tunnel: w1490 -> [w1501]
                  tunnel: w1489 -> [w1500]
                  tunnel: w1488 -> [w1499]
                  tunnel: w1487 -> [w1498]
                  n541 = case shown="\"m4_5_0\"" w1502 {
                    selector: w1502 -> [_ w1507 w1511 w1515 w1519]
                    tunnel: w1504 -> [w1505 w1509 w1513 w1517 w1521]
                    tunnel: [w1505 w1508 w1512 w1516 w1520] -> w1503
                    tunnel: w1501 -> [_ w1506 _ _ _]
                    tunnel: w1500 -> [_ _ w1510 _ _]
                    tunnel: w1499 -> [_ _ _ w1514 _]
                    tunnel: w1498 -> [_ _ _ _ w1518]
                    frame "假", Default {
                    }
                    frame "m4_5_3" {
                      n542 = Set Menu Item Info(6:w1506, 7:w1507, 11:w1509) -> (3:w1508:refnum<k9>)  [unwired: 4 in, 1 out]
                    }
                    frame "m4_5_2" {
                      n543 = Set Menu Item Info(6:w1510, 7:w1511, 11:w1513) -> (3:w1512:refnum<k9>)  [unwired: 4 in, 1 out]
                    }
                    frame "m4_5_1" {
                      n544 = Set Menu Item Info(6:w1514, 7:w1515, 11:w1517) -> (3:w1516:refnum<k9>)  [unwired: 4 in, 1 out]
                    }
                    frame "m4_5_0" {
                      n545 = Set Menu Item Info(6:w1518, 7:w1519, 11:w1521) -> (3:w1520:refnum<k9>)  [unwired: 4 in, 1 out]
                    }
                  }
                }
                n546 = Format Into String(format string="数据格式(%s)" ("格式字符串"), w1474) -> (resulting string=w1479:string)  [unwired: 2 in, 1 out]
                n547 = invoke class="VI" method="Ctrl Val.Set"(reference=w1478, "Control Name"="ForceUpt" ("控件名"), "Value"=TRUE) -> ()  [unwired: 2 in, 5 out]
                n548 = Bundle By Name(cluster=w1494, "format"=w1474) -> (w1493:T2)
                n549 = Set Menu Item Info(7:"m4_5" ("项标识符"), 10:w1479, 11:w1481) -> ()  [unwired: 4 in, 2 out]
              }
              frame "m4_6_0" {
                n550 = Get Menu Item Info(7:w1555, 11:w1556) -> (3:w1558:refnum<k9>, 4:w1557:bool)  [unwired: 1 in, 5 out]
                n551 = Not(x=w1557) -> (.not. x?=w1545:bool)
                n552 = Set Menu Item Info(6:w1545, 7:w1555, 11:w1558) -> ()  [unwired: 4 in, 2 out]
                n553 = invoke class="VI" method="Ctrl Val.Set"(reference=w1554, "Control Name"="Rrate1" ("控件名"), "Value"=w1545) -> ()  [unwired: 2 in, 5 out]
                n554 = property on="Rrate1" class="DigNum (严格)"() -> ("Value"=w1544:dbl)  [unwired: 2 in, 2 out]
                n555 = Select(t=T4."Enabled" ("禁用"), s=w1545, f=T4."Disabled and Grayed Out" ("禁用")) -> (s? t:f=w1546:T4)
                n556 = Bundle By Name(cluster=w1551, "rateR1"=w1545) -> (w1552:T2)
                n557 = Select(t=w1544, s=w1545, f=0.0) -> (s? t:f=w1542:dbl)
                n558 = property on="Rrate1" class="DigNum (严格)"("DisabledEnum"=w1546, "Value"=w1542) -> ()  [unwired: 2 in, 2 out]
              }
              frame "m4_6_1" {
                n559 = Get Menu Item Info(7:w1579, 11:w1580) -> (3:w1582:refnum<k9>, 4:w1581:bool)  [unwired: 1 in, 5 out]
                n560 = Not(x=w1581) -> (.not. x?=w1564:bool)
                n561 = Set Menu Item Info(6:w1564, 7:w1579, 11:w1582) -> ()  [unwired: 4 in, 2 out]
                n562 = Unbundle By Name(w1563) -> ("type"=w1567:u16)
                n563 = Equal?(x=u16 4, y=w1567) -> (x = y?=w1565:bool)
                n564 = property on="Rrate2" class="DigNum (严格)"() -> ("Value"=w1570:dbl)  [unwired: 2 in, 2 out]
                n565 = And(x=w1565, y=w1564) -> (x .and. y?=w1562:bool)
                n566 = invoke class="VI" method="Ctrl Val.Set"(reference=w1578, "Control Name"="Rrate2" ("控件名"), "Value"=w1562) -> ()  [unwired: 2 in, 5 out]
                n567 = Bundle By Name(cluster=w1563, "rateR2"=w1564) -> (w1576:T2)
                n568 = Select(t=w1570, s=w1562, f=0.0) -> (s? t:f=w1568:dbl)
                n569 = Select(t=T4."Enabled" ("禁用"), s=w1562, f=T4."Disabled and Grayed Out" ("禁用")) -> (s? t:f=w1571:T4)
                n570 = property on="Rrate2" class="DigNum (严格)"("DisabledEnum"=w1571, "Value"=w1568) -> ()  [unwired: 2 in, 2 out]
              }
              frame "m4_7_0" {
                n571 = Get Menu Item Info(7:w1599, 11:w1600) -> (3:w1602:refnum<k9>, 4:w1601:bool)  [unwired: 1 in, 5 out]
                n572 = Not(x=w1601) -> (.not. x?=w1589:bool)
                n573 = Set Menu Item Info(6:w1589, 7:w1599, 11:w1602) -> ()  [unwired: 4 in, 2 out]
                n574 = invoke class="VI" method="Ctrl Val.Set"(reference=w1598, "Control Name"="Trate1" ("控件名"), "Value"=w1589) -> ()  [unwired: 2 in, 5 out]
                n575 = property on="Trate1" class="DigNum (严格)"() -> ("Value"=w1588:dbl)  [unwired: 2 in, 2 out]
                n576 = Select(t=T4."Enabled" ("禁用"), s=w1589, f=T4."Disabled and Grayed Out" ("禁用")) -> (s? t:f=w1590:T4)
                n577 = Bundle By Name(cluster=w1595, "rateT1"=w1589) -> (w1596:T2)
                n578 = Select(t=w1588, s=w1589, f=0.0) -> (s? t:f=w1586:dbl)
                n579 = property on="Trate1" class="DigNum (严格)"("DisabledEnum"=w1590, "Value"=w1586) -> ()  [unwired: 2 in, 2 out]
              }
              frame "m4_7_1" {
                n580 = Get Menu Item Info(7:w1623, 11:w1624) -> (3:w1626:refnum<k9>, 4:w1625:bool)  [unwired: 1 in, 5 out]
                n581 = Not(x=w1625) -> (.not. x?=w1608:bool)
                n582 = Set Menu Item Info(6:w1608, 7:w1623, 11:w1626) -> ()  [unwired: 4 in, 2 out]
                n583 = Unbundle By Name(w1607) -> ("type"=w1611:u16)
                n584 = Equal?(x=u16 4, y=w1611) -> (x = y?=w1609:bool)
                n585 = property on="Trate2" class="DigNum (严格)"() -> ("Value"=w1614:dbl)  [unwired: 2 in, 2 out]
                n586 = And(x=w1609, y=w1608) -> (x .and. y?=w1606:bool)
                n587 = invoke class="VI" method="Ctrl Val.Set"(reference=w1622, "Control Name"="Trate2" ("控件名"), "Value"=w1606) -> ()  [unwired: 2 in, 5 out]
                n588 = Bundle By Name(cluster=w1607, "rateT2"=w1608) -> (w1620:T2)
                n589 = Select(t=w1614, s=w1606, f=0.0) -> (s? t:f=w1612:dbl)
                n590 = Select(t=T4."Enabled" ("禁用"), s=w1606, f=T4."Disabled and Grayed Out" ("禁用")) -> (s? t:f=w1615:T4)
                n591 = property on="Trate2" class="DigNum (严格)"("DisabledEnum"=w1615, "Value"=w1612) -> ()  [unwired: 2 in, 2 out]
              }
              frame "m5_0" {
                w1631 = "\r\n"
                n592 = call "USB_CAN_VerInfo.vi"() -> ("VerInfo"=w1633:string)  [unwired: 11 in]
                n593 = Concatenate Strings("USB-CAN Tool V" ("Infoin"), w1630, w1631, w1633, w1631, w1631, "创芯光电科技有限公司，版权所有2013" ("Infoin")) -> (w1634:string)
                n594 = call "USB_CAN_ABOUT_DLG.vi"("Info"=w1634, "Title"="关于USB-CAN Tool" ("title")) -> ()  [unwired: 10 in]
              }
            }
          }
          event User Event {
            n595 = event-data() -> ("openCan"=w1654:bool)  [unwired: 1 in]
            n596 = call "FindUSBDevice.vi"("DevSNin"="") -> ("DevSN"=w1643:string, "DevNum"=w1645:i32)  [unwired: 6 in, 3 out]
            n597 = case shown="0.." w1645 {
              selector: w1645 -> [_ w1677]
              tunnel: [_ w1694] -> w1658
              tunnel: ["提示" ("title") w1693] -> w1656
              tunnel: ["打开失败！" ("Infoin") w1692] -> w1655
              tunnel: w1653 -> [w1671 w1691]
              tunnel: [w1671 w1690] -> w1652
              tunnel: w1651 -> [w1670 w1689]
              tunnel: w1650 -> [_ w1688]
              tunnel: [w1670 w1687] -> w1649
              tunnel: [w1673 w1680] -> w1648
              tunnel: w1647 -> [_ w1679]
              tunnel: w1644 -> [w1673 _]
              tunnel: w1643 -> [_ w1676]
              frame -1, Default {
              }
              frame 0.. {
                n598 = call "PreOpenDevice.vi"("Index"=w1677, "type"=w1679, "param"=w1689) -> ("Channels"=w1678:u32[], "DevIndex"=w1680:u32, "param out"=w1687:T5[])  [unwired: 6 in]
                n599 = Unbundle By Name(w1688) -> ("RcvLen"=w1675:i16, "RcvE1"=w1686:bool, "RcvE2"=w1683:bool, "type"=w1685:u16)
                n600 = Equal?(x=w1685, y=u16 4) -> (x = y?=w1681:bool)
                n601 = And(x=w1683, y=w1681) -> (x .and. y?=w1682:bool)
                n602 = call "OpenDevice.vi"("RcvLen"=w1675, "Enable2"=w1682, "DevIndex"=w1680, "Enable1"=w1686, "param"=w1687, "Channels"=w1678, "type"=w1679) -> ("open"=w1694:bool)  [unwired: 3 in, 1 out]
                n603 = case shown="真" w1694 {
                  tunnel: ["提示信息" ("title") "提示" ("title")] -> w1693
                  tunnel: ["USB-CAN设备打开失败！" ("Infoin") "USB-CAN设备打开成功！" ("Infoin")] -> w1692
                  tunnel: w1691 -> [w1695 w1708]
                  tunnel: [w1695 w1707] -> w1690
                  tunnel: w1679 -> [_ w1706]
                  tunnel: w1676 -> [_ w1699]
                  frame False {
                  }
                  frame True {
                    w1700 = " - " ("字符串")
                    n604 = Equal?(x=w1706, y=u16 4) -> (x = y?=w1704:bool)
                    n605 = Select(t="USB_CAN2" ("字符串"), s=w1704, f="USB_CAN" ("字符串")) -> (s? t:f=w1701:string)
                    n606 = Concatenate Strings(w1708, w1700, w1701, w1700, "SN:" ("字符串"), w1699) -> (w1707:string)
                  }
                }
              }
            }
            "DevIndex" <- w1648
            n607 = global write "_USB_CAN_GLOBAL_.vi" "open"(w1658) -> ()
            n608 = property class="VI"("Front Panel.Title"=w1652) -> ()  [unwired: 2 in, 2 out]
            n609 = case shown="真" w1654 {
              tunnel: w1656 -> [_ w1712]
              tunnel: w1655 -> [_ w1711]
              frame False {
              }
              frame True {
                n610 = call "TimeLmtDialog.vi"("Infoin"=w1711, "title"=w1712) -> ()  [unwired: 10 in]
              }
            }
          }
          event Panel Close? {
            n611 = event-data() -> ()  [unwired: 1 in, 1 out]
            n612 = event-data("Discard?"=TRUE ("放弃？")) -> ()  [unwired: 1 in, 1 out]
          }
          event "sendfile": Value Change {
            n613 = event-data() -> ()  [unwired: 1 in, 1 out]
            n614 = case shown="真" w1734 {
              tunnel: w1736 -> [_ w1769]
              tunnel: w1731 -> [_ w1751]
              frame False {
                n615 = call "TimeLmtDialog.vi"("Infoin"="USB-CAN设备未打开！", "title"="提示") -> ()  [unwired: 10 in]
              }
              frame True {
                n616 = invoke class="VI" method="Ctrl Val.Set"(reference=w1769, "Control Name"="sendfile" ("控件名"), "Value"=TRUE) -> (reference out=w1765:refnum<vi>, error out=w1759:errorcluster)  [unwired: 2 in, 3 out]
                n617 = local read "SendCnt"() -> (w1762:i32)
                n618 = invoke class="VI" method="Ctrl Val.Set"(reference=w1765, error in=w1759, "Control Name"="FrameCnt" ("控件名"), "Value"=w1762) -> (reference out=w1761:refnum<vi>, error out=w1760:errorcluster)  [unwired: 1 in, 3 out]
                n619 = local read "sendcycle"() -> (w1755:i32)
                n620 = invoke class="VI" method="Ctrl Val.Set"(reference=w1761, error in=w1760, "Control Name"="Cycle" ("控件名"), "Value"=w1755) -> (reference out=w1757:refnum<vi>, error out=w1758:errorcluster)  [unwired: 1 in, 3 out]
                n621 = invoke class="VI" method="Ctrl Val.Set"(reference=w1757, error in=w1758, "Control Name"="Enable" ("控件名"), "Value"=TRUE) -> (reference out=w1754:refnum<vi>, error out=w1753:errorcluster)  [unwired: 1 in, 3 out]
                n622 = invoke class="VI" method="Ctrl Val.Set"(reference=w1754, error in=w1753, "Control Name"="channel" ("控件名"), "Value"=w1751) -> ()  [unwired: 1 in, 5 out]
              }
            }
          }
          event "savefile": Value Change {
            w1770 = TRUE
            n623 = event-data() -> ()  [unwired: 1 in, 1 out]
            n624 = invoke class="VI" method="Ctrl Val.Set"(reference=w1778, "Control Name"="save" ("控件名"), "Value"=w1770) -> (reference out=w1772:refnum<vi>, error out=w1771:errorcluster)  [unwired: 2 in, 3 out]
            n625 = invoke class="VI" method="Ctrl Val.Set"(reference=w1772, error in=w1771, "Control Name"="sPth_Sel" ("控件名"), "Value"=w1770) -> ()  [unwired: 1 in, 5 out]
            n626 = Set Menu Item Info(6:w1770, 7:"m4_2" ("控件名"), 11:w1774) -> ()  [unwired: 4 in, 2 out]
            n627 = Bundle By Name(cluster=w1776, "save"=w1770) -> (w1775:T2)
            n628 = property on="path" class="Path"("Value"=path "" ("path")) -> ()  [unwired: 2 in, 2 out]
          }
          event "clear": Value Change {
            n629 = event-data() -> ()  [unwired: 1 in, 1 out]
            n630 = invoke class="VI" method="Ctrl Val.Set"(reference=w1802, "Control Name"="clear" ("控件名"), "Value"=TRUE) -> ()  [unwired: 2 in, 5 out]
          }
          event "reciveEnable": Value Change {
            n631 = event-data() -> ("NewVal"=w1817:bool)  [unwired: 1 in]
            n632 = invoke class="VI" method="Ctrl Val.Set"(reference=w1823, "Control Name"="Enable" ("控件名"), "Value"=w1817) -> ()  [unwired: 2 in, 5 out]
            n633 = global write "_USB_CAN_GLOBAL_.vi" "R-Enb"(w1817) -> ()
          }
          event "Send": Value Change {
            n634 = event-data() -> ()  [unwired: 1 in, 1 out]
            n635 = case shown="真" w1841 {
              tunnel: w1846 -> [_ w1861]
              tunnel: w1845 -> [_ w1860]
              tunnel: w1844 -> [_ w1859]
              tunnel: w1843 -> [_ w1858]
              tunnel: w1837 -> [_ w1857]
              frame False {
                n636 = call "TimeLmtDialog.vi"("Infoin"="USB-CAN设备未打开！", "title"="提示") -> ()  [unwired: 10 in]
              }
              frame True {
                w1863 = T4."Disabled and Grayed Out" ("禁用")
                n637 = property on="send stop" class="Bool (严格)"("DisabledEnum"=T4."Enabled" ("禁用")) -> ()  [unwired: 2 in, 2 out]
                n638 = property on="Send" class="Bool"("DisabledEnum"=w1863) -> ()  [unwired: 2 in, 2 out]
                n639 = property on="data" class="Str"("DisabledEnum"=w1863) -> ()  [unwired: 2 in, 2 out]
                n640 = property on="ID Inc" class="Bool (严格)"("DisabledEnum"=w1863) -> ()  [unwired: 2 in, 2 out]
                n641 = property on="sendcycle" class="DigNum (严格)"("DisabledEnum"=w1863) -> ()  [unwired: 2 in, 2 out]
                n642 = property on="Data Inc" class="Bool (严格)"("DisabledEnum"=w1863) -> ()  [unwired: 2 in, 2 out]
                n643 = property on="SendCnt" class="DigNum (严格)"("DisabledEnum"=w1863) -> ()  [unwired: 2 in, 2 out]
                n644 = for {
                  N: 10 -> [_]
                  tunnel: w1861 -> [w1869]
                  tunnel: w1860 -> [w1868]
                  tunnel: w1859 -> [w1867]
                  tunnel: w1858 -> [w1866]
                  tunnel: w1857 -> [w1865]
                  i -> [w1870]
                  n645 = case shown="9" w1870 {
                    tunnel: w1869 -> [_ w1873 w1876 w1879 w1882 w1885 w1888 w1892 w1896 w1899 w1902]
                    tunnel: w1868 -> [_ w1871 _ _ _ _ _ _ _ _ _]
                    tunnel: w1867 -> [_ _ w1874 _ _ _ _ _ _ _ _]
                    tunnel: w1866 -> [_ _ _ _ _ _ w1886 _ _ _ _]
                    tunnel: w1865 -> [_ _ _ _ _ _ _ _ _ _ w1900]
                    frame -1, Default {
                    }
                    frame 0 {
                      n646 = invoke class="VI" method="Ctrl Val.Set"(reference=w1873, "Control Name"="data" ("控件名"), "Value"=w1871) -> ()  [unwired: 2 in, 5 out]
                    }
                    frame 1 {
                      n647 = invoke class="VI" method="Ctrl Val.Set"(reference=w1876, "Control Name"="FrameCnt" ("控件名"), "Value"=w1874) -> ()  [unwired: 2 in, 5 out]
                    }
                    frame 2 {
                      n648 = invoke class="VI" method="Ctrl Val.Set"(reference=w1879, "Control Name"="Cycle" ("控件名"), "Value"="sendcycle") -> ()  [unwired: 2 in, 5 out]
                    }
                    frame 3 {
                      n649 = invoke class="VI" method="Ctrl Val.Set"(reference=w1882, "Control Name"="ID Inc" ("控件名"), "Value"="ID Inc") -> ()  [unwired: 2 in, 5 out]
                    }
                    frame 4 {
                      n650 = invoke class="VI" method="Ctrl Val.Set"(reference=w1885, "Control Name"="Data Inc" ("控件名"), "Value"="Data Inc") -> ()  [unwired: 2 in, 5 out]
                    }
                    frame 5 {
                      n651 = invoke class="VI" method="Ctrl Val.Set"(reference=w1888, "Control Name"="ID" ("控件名"), "Value"=w1886) -> ()  [unwired: 2 in, 5 out]
                    }
                    frame 6 {
                      n652 = local read "Frame Format"() -> (w1890:enum16{"标准帧", "扩展帧"})
                      n653 = Not Equal To 0?(x=w1890) -> (x != 0?=w1889:bool)
                      n654 = invoke class="VI" method="Ctrl Val.Set"(reference=w1892, "Control Name"="ExtFrame" ("控件名"), "Value"=w1889) -> ()  [unwired: 2 in, 5 out]
                    }
                    frame 7 {
                      n655 = local read "Frame Type"() -> (w1893:enum16{"数据帧", "远程帧"})
                      n656 = Not Equal To 0?(x=w1893) -> (x != 0?=w1894:bool)
                      n657 = invoke class="VI" method="Ctrl Val.Set"(reference=w1896, "Control Name"="remote" ("控件名"), "Value"=w1894) -> ()  [unwired: 2 in, 5 out]
                    }
                    frame 8 {
                      n658 = invoke class="VI" method="Ctrl Val.Set"(reference=w1899, "Control Name"="Enable" ("控件名"), "Value"=TRUE) -> ()  [unwired: 2 in, 5 out]
                    }
                    frame 9 {
                      n659 = invoke class="VI" method="Ctrl Val.Set"(reference=w1902, "Control Name"="channel" ("控件名"), "Value"=w1900) -> ()  [unwired: 2 in, 5 out]
                    }
                  }
                }
              }
            }
          }
          event "send stop": Value Change {
            w1905 = FALSE
            w1913 = T4."Enabled" ("禁用")
            n660 = event-data() -> ()  [unwired: 1 in, 1 out]
            n661 = Not(x=w1905) -> (.not. x?=w1904:bool)
            n662 = invoke class="VI" method="Ctrl Val.Set"(reference=w1909, "Control Name"="Enable" ("控件名"), "Value"=w1905) -> ()  [unwired: 2 in, 5 out]
            n663 = global write "_USB_CAN_GLOBAL_.vi" "S-Cancel"(w1904) -> ()
            n664 = property on="send stop" class="Bool (严格)"("DisabledEnum"=T4."Disabled and Grayed Out" ("禁用")) -> ()  [unwired: 2 in, 2 out]
            n665 = property on="Send" class="Bool"("DisabledEnum"=w1913) -> ()  [unwired: 2 in, 2 out]
            n666 = property on="data" class="Str"("DisabledEnum"=w1913) -> ()  [unwired: 2 in, 2 out]
            n667 = property on="ID Inc" class="Bool (严格)"("DisabledEnum"=w1913) -> ()  [unwired: 2 in, 2 out]
            n668 = property on="sendcycle" class="DigNum (严格)"("DisabledEnum"=w1913) -> ()  [unwired: 2 in, 2 out]
            n669 = property on="Data Inc" class="Bool (严格)"("DisabledEnum"=w1913) -> ()  [unwired: 2 in, 2 out]
            n670 = property on="SendCnt" class="DigNum (严格)"("DisabledEnum"=w1913) -> ()  [unwired: 2 in, 2 out]
            n671 = local write "send stop"(FALSE ("send stop")) -> ()
          }
          event "ID Filter Set": Value Change {
            n672 = event-data() -> ()  [unwired: 1 in, 1 out]
            n673 = call "str_to_u32_arr.vi"("string"="ID Filter Str") -> ("array"=w1927:u32[])
            n674 = Select(t=w1927, s=w1939, f=w1942) -> (s? t:f=w1937:u32[])
            n675 = invoke class="VI" method="Ctrl Val.Set"(reference=w1932, "Control Name"="UseFilter" ("控件名"), "Value"=TRUE) -> (reference out=w1933:refnum<vi>)  [unwired: 2 in, 4 out]
            n676 = invoke class="VI" method="Ctrl Val.Set"(reference=w1933, "Control Name"="Filter" ("控件名"), "Value"=w1937) -> ()  [unwired: 2 in, 5 out]
          }
          event "ID Filter": Value Change {
            n677 = event-data() -> ("NewVal"=w1965:enum32{"enable", "disable"})  [unwired: 1 in]
            n678 = Equal?(x=w1965, y=enum32{"enable", "disable"}."enable") -> (x = y?=w1955:bool)
            n679 = Select(t=T4."Enabled" ("禁用"), s=w1955, f=T4."Disabled and Grayed Out" ("禁用")) -> (s? t:f=w1961:T4)
            n680 = property on="ID Filter Str" class="Str"("DisabledEnum"=w1961) -> ()  [unwired: 2 in, 2 out]
            n681 = property on="ID Filter Set" class="Bool"("DisabledEnum"=w1961) -> ()  [unwired: 2 in, 2 out]
            n682 = case shown="假" w1955 {
              selector: w1955 -> [w1975 _]
              tunnel: w1958 -> [w1979 _]
              tunnel: w1957 -> [w1976 _]
              frame False {
                n683 = invoke class="VI" method="Ctrl Val.Set"(reference=w1979, "Control Name"="UseFilter" ("控件名"), "Value"=w1975) -> (reference out=w1977:refnum<vi>)  [unwired: 2 in, 4 out]
                n684 = invoke class="VI" method="Ctrl Val.Set"(reference=w1977, "Control Name"="Filter" ("控件名"), "Value"=w1976) -> ()  [unwired: 2 in, 5 out]
              }
              frame True {
              }
            }
          }
          event "ID Type": Value Change {
            n685 = event-data() -> ("NewVal"=w1987:enum32{"left", "right"})  [unwired: 1 in]
          }
          event "data": Value Change {
            n686 = event-data() -> ("NewVal"=w2003:string)  [unwired: 1 in]
            n687 = call "str_to_u32_arr.vi"("string"=w2003) -> ("array"=w2002:u32[])
            n688 = To Unsigned Byte Integer(number=w2002) -> (unsigned 8bit integer=w2001:u8[])
          }
          event "SendCnt": Value Change {
            n689 = event-data() -> ("NewVal"=w2023:i32)  [unwired: 1 in]
          }
          event "CAN Channel": Value Change {
            n690 = event-data() -> ("NewVal"=w2040:enum16{"1", "2"})  [unwired: 1 in]
          }
          event "Frame ID": Value Change {
            n691 = event-data() -> ("NewVal"=w2058:string)  [unwired: 1 in]
            n692 = call "FormatIDString.vi"("ID String"=w2058) -> ("ID"=w2057:u32)
          }
          event "Frame Type": Value Change {
            n693 = event-data() -> ("NewVal"=w2075:enum16{"数据帧", "远程帧"})  [unwired: 1 in]
          }
          event "Frame Format": Value Change {
            n694 = event-data() -> ("NewVal"=w2092:enum16{"标准帧", "扩展帧"})  [unwired: 1 in]
          }
        }
      }
      frame "unRegistEvent" {
        n695 = local read "DevIndex"() -> (w2104:u32)
        n696 = stacked-sequence {
          tunnel: w2103 -> [w2130 w2140]
          tunnel: w2104 -> [w2129 w2139]
          frame #0 {
            n697 = Equal?(x=w2130, y=u16 4) -> (x = y?=w2134:bool)
            n698 = Select(t=2, s=w2134, f=1) -> (s? t:f=w2131:i32)
            n699 = for {
              N: w2131 -> [_]
              tunnel: w2130 -> [w2138]
              tunnel: w2129 -> [w2137]
              i -> [w2136]
              n700 = call "ResetCAN.vi"("CANInd"=w2136, "DeciceInd"=w2137, "DeviceType"=w2138) -> ()  [unwired: 7 in, 2 out]
            }
          }
          frame #1 {
            n701 = call "CloseDevice.vi"("DeviceInd"=w2139, "type"=w2140) -> ()  [unwired: 8 in, 2 out]
          }
        }
        n702 = Unregister For Events(event registration refnum=w2117) -> (error out=w2116:errorcluster)  [unwired: 1 in]
        n703 = Destroy User Event(user event=w2115, error in=w2116) -> (error out=w2113:errorcluster)
        n704 = call "_USB_CAN_PARAM_RW_.vi"("write"=TRUE, "param"=w2111) -> ()  [unwired: 9 in, 1 out]
        n705 = Destroy User Event(user event=w2112, error in=w2113) -> (error out=w2107:errorcluster)
        n706 = Destroy User Event(user event=w2106, error in=w2107) -> ()  [unwired: 1 out]
        n707 = property class="VI"(reference=w2120) -> (reference out=w2122:refnum<vi>, "Exec.State"=w2121:T8)  [unwired: 1 in, 1 out]
        n708 = property class="VI"(reference=w2127) -> (reference out=w2125:refnum<vi>, "Exec.State"=w2126:T8)  [unwired: 1 in, 1 out]
        n709 = case shown="\"Run top level\", \"Running\"" w2121 {
          tunnel: w2122 -> [w2141 w2146]
          tunnel: [w2141 w2145] -> w2123
          frame "Bad", Default {
          }
          frame "Run top level", "Running" {
            n710 = invoke class="VI" method="Ctrl Val.Set"(reference=w2146, "Control Name"="stop" ("控件名"), "Value"=TRUE) -> (reference out=w2145:refnum<vi>, error out=w2142:errorcluster)  [unwired: 2 in, 3 out]
            n711 = call "0.1秒"("error in (no error)"=w2142) -> ()  [unwired: 10 in, 1 out]
          }
        }
        n712 = case shown="\"Run top level\", \"Running\"" w2126 {
          tunnel: w2125 -> [w2147 w2152]
          tunnel: [w2147 w2151] -> w2124
          frame "Bad", Default {
          }
          frame "Run top level", "Running" {
            n713 = invoke class="VI" method="Ctrl Val.Set"(reference=w2152, "Control Name"="stop" ("控件名"), "Value"=TRUE) -> (reference out=w2151:refnum<vi>, error out=w2148:errorcluster)  [unwired: 2 in, 3 out]
            n714 = call "0.1秒"("error in (no error)"=w2148) -> ()  [unwired: 10 in, 1 out]
          }
        }
        n715 = Close Reference(reference=w2123) -> ()  [unwired: 1 in, 1 out]
        n716 = Close Reference(reference=w2124) -> (error out=w2114:errorcluster)  [unwired: 1 in]
        n717 = global write "_USB_CAN_GLOBAL_.vi" "R-Enable"(FALSE ("R-Enable")) -> ()
        n718 = global write "_USB_CAN_GLOBAL_.vi" "S-Enable"(FALSE ("R-Enable")) -> ()
      }
      frame "Release" {
        n719 = call "ReciveBuffer.vi"("销毁?"=TRUE) -> ()  [unwired: 1 out]
        n720 = call "MonitorBuffer.vi"("销毁?"=TRUE) -> ()  [unwired: 1 out]
        n721 = call "SendBuffer.vi"("销毁"=TRUE) -> ()  [unwired: 1 out]
        n722 = control-ref of="本VI"() -> (w2155:refnum<vi>)
        n723 = call "UI_Status.vi"("write?"=TRUE, "menu status in"=w2154, "VI ref"=w2155) -> ()  [unwired: 7 in, 2 out]
      }
      frame "Exit" {
      }
    }
  }
  n724 = control-ref of="本VI"() -> (w2:refnum<vi>)
  n725 = call "Exit.vi"("error in (no error)"=w3, "VI引用"=w2) -> ()  [unwired: 9 in, 1 out]
